vi "XY_plot_gnuplot.vi"(0 "Plot Array":cluster{dbl[], dbl[]}[](array[cluster])=[{[500.0, 500.0, 953.54, 215.0, 270.0, 320.0, 445.0, 525.0, 600.0, 675.0, 750.0, 825.0, 900.0, 960.0, 1010.0, 1060.0], [4.614524, 4.54365, 5.818368, 0.1374656, 0.6662545, 1.465458, 3.619824, 4.848976, 5.887329, 5.940571, 6.152151, 5.717487, 5.600293, 5.40069, 5.154843, 5.121789]}, {[100.0, 150.0, 215.0, 270.0, 320.0, 445.0, 525.0, 600.0, 675.0, 750.0, 825.0, 900.0, 960.0, 1010.0, 1060.0], [0.002314715, -0.00693192, 0.120417, 0.6880509, 1.519176, 3.513709, 5.065183, 6.116033, 6.096773, 5.938465, 5.593788, 5.5597, 5.387002, 5.304077, 4.887903]}] {"?" format="%.2f"; "?" format="%.2f"}, 1 "Job Directory":path=path "/G4_2_HD/Users/paulhayden/Documents/Projects/Westlakes_resolution") -> (2 "Saved Automatically?":bool, 3 "Tex Info String":string="set term epslatex\nset output \"Plot.eps\"\nset xlabel '$Distance~(m)$'\nset ylabel '$DF~(s/m^3)\\times10^6$'\nset samples 1000\nset pointsize 1.00\nset title '$B38~Centreline~Glc$' 0, 0\nset size 0.75,0.9\n\n#set key 450, -2.5833\n unset key\nset label 1 '~~~~~~~~~~~Angle~(deg)~=~0' at -100, -2.58\nset label 2 '~~~~~~~~~~~Height~(m)~=~5' at -100, -3.27\n set xrange [0 : 500] \n# set autoscale x \n set yrange [0.10000 : 7]\n# set autoscale y \n\nplot \"B38_Centreline_Glc.dat\" index 0 using 1:2 axes x1y1 title '$File=B38R~DDD.xls$' with points 1 1, \\\n\"B38_Centreline_Glc.dat\" index 1 using 1:2 axes x1y1 title '$File=B38R~DDD~1.xls$' with points 1 3", 4 "Plot data file":path)   [LabVIEW 2012]
uses:
  Gnuplot_Label.ctl
  gnuplotScriptComponents/gridlines.ctl
  gnuplotScriptComponents/legendProperties.ctl
  gnuplotScriptComponents/legendAppearance.ctl
  gnuplotScriptComponents/alignment.ctl
  gnuplotScriptComponents/at.ctl
  Results_plotter_Global.vi
  <vilib>/Analysis/baseanly.llb/Mean (DBL).vi
  <vilib>/Analysis/NI_AALBase.lvlib
  <vilib>/Analysis/NI_AALPro.lvlib
panel:
  in  "Call GNUPLOT":bool
  in  "Show Re-Run Gnuplot?":bool
  in  "Tab Control":T1(tab)
  in  "Plot Title":u16(ring) items=["Title String Only", "Number of Measurements", "WD::", "Pt::", "U0:W:", "U1:W:", "U2:W:l", "U2:W:u", "U3:W:", "U4:W:", "U0:E:", "U1:E:", "U2:E:l", "U2:E:u", "U3:E:", "U4:E:", "U2_{tower}::", "U3_{tower}::", "U4_{tower}::", "U3W/U3_{tower}::", "U3E/U3_{tower}::", "U4W/U4_{tower}::", "U4E/U4_{tower}::", "U0W/U4W::", "U0E/U4E::", "$U0W/U4_{tower}$::", "$U0E/U4_{tower}$::", "U2Wl/U2_{tower}::", "U2Wu/U2_{tower}::", "U2El/U2_{tower}::", "U2Eu/U2_{tower}::"]
  in  "Plot Title":string
  in  "Added labels":i32[](listbox)
  in  "Show Labels?":bool
  in  "Summarise":u16(ring) items=["All Series", "U2Wl/U2_{tower}__Pt=1__", "U2Wl/U2_{tower}__Pt=2__", "U2Wl/U2_{tower}__Pt=3__", "U2Wl/U2_{tower}__Pt=4__", "U2Wu/U2_{tower}__Pt=1__", "U2Wu/U2_{tower}__Pt=2__", "U2Wu/U2_{tower}__Pt=3__", "U2Wu/U2_{tower}__Pt=4__"]
  in  "X Log?":bool
  in  "Y Log?":bool
  in  "Ymin Val":dbl
  in  "Ymin":bool=TRUE
  in  "Xmin Val":dbl
  in  "Xmin":bool=TRUE
  in  "Xmax Val":dbl
  in  "Xmax":bool=TRUE
  in  "Ymax Val":dbl
  in  "Ymax":bool=TRUE
  in  "Major Gridlines":T2
  in  "Minor Gridlines":T2
  out "Time format?":bool
  in  "precision":string
  out "Profile offset":dbl
  in  "Offset?":bool
  in  "Mode":T3
  in  "Separation":dbl=1.2
  in  "Fit type":T4(ring)
  in  "Put Coeff\nin Results file":bool
  in  "Analysis":T5(ring)
  in  "Wavelength?":bool
  in  "Auto Zp":bool=TRUE
  in  "Fixed Zp":dbl format="%.2f"
  in  "Something about fit..!":bool
  in  "Black and white?":bool
  in  "plot error bars?":bool
  in  "Plot style":u16[](array[ring])=[0, 0, 0, 0, 0, 0, 0, 0, 0, 0, 0] items=["points", "lines", "linespoints"]
  in  "Point Size":dbl=1.2 format="%.2f"
  in  "Graph Height":string="0.9"
  in  "Graph width":string="0.75"
  in  "Show legend?":bool
  in  "Legend Position":u16(ring) items=["LabVIEW calculated", "top left", "top right", "bottom left", "bottom right", "below"]
  in  "Reverse order":bool
  in  "Save data analysis file":bool
  out "Path":path
  in  "Filename Max length":i32=28
  out "With legend":i32=580
  out "No Legend":i32=397
  out "No of Series":i32=2
  out "X location":dbl=-100.0
  out "Y location":dbl=-2.583333333333333
  out "Delta y":dbl=0.6900000000000001
  out "Extra range":dbl
  out "Final Title":string="B38 Centreline Glc"
  out "XY Graph":cluster{dbl[], dbl[]}[](graph)=[{[215.0, 270.0, 320.0, 445.0, 500.0, 500.0, 525.0, 600.0, 675.0, 750.0, 825.0, 900.0, 953.54, 960.0, 1010.0, 1060.0], [0.1374656, 0.6662545, 1.465458, 3.619824, 4.614524, 4.54365, 4.848976, 5.887329, 5.940571, 6.152151, 5.717487, 5.600293, 5.818368, 5.40069, 5.154843, 5.121789]}, {[100.0, 150.0, 215.0, 270.0, 320.0, 445.0, 525.0, 600.0, 675.0, 750.0, 825.0, 900.0, 960.0, 1010.0, 1060.0], [0.002314715, -0.00693192, 0.120417, 0.6880509, 1.519176, 3.513709, 5.065183, 6.116033, 6.096773, 5.938465, 5.593788, 5.5597, 5.387002, 5.304077, 4.887903]}]
  # "Scales"
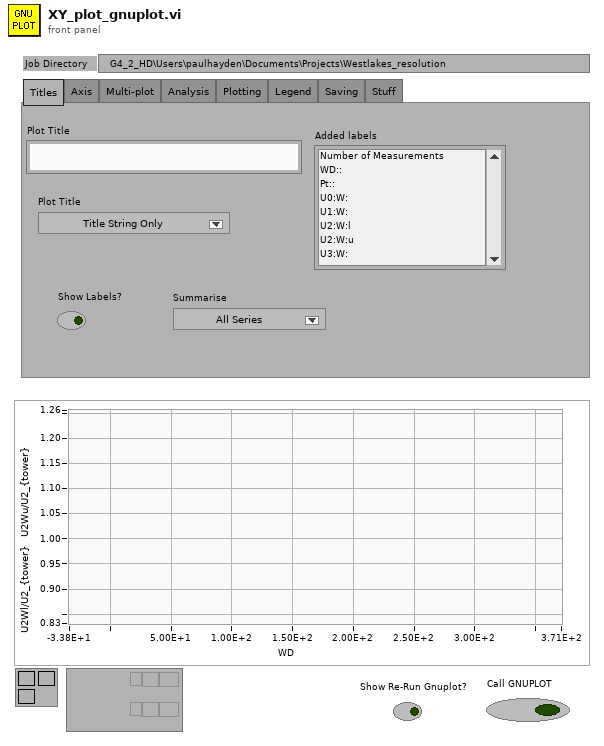
[diagram p1: front panel]
types:
  T1 = enum32{"Titles", "Axis", "Multi-plot", "Analysis", "Plotting", "Legend", "Saving", "Stuff"}
  T2 = typedef "gridlines.ctl" = enum16{"None", "X only", "Y only", "Both X and Y"}
  T3 = typedef "Gnuplot_Label.ctl" = enum16{"3 Labels per plot", "Only Center label", "Only Bottom Label"}
  T4 = enum16{"None", "Spline", "Linear", "2nd Poly", "3rd Poly", "4th Poly", "Gauss Lat", "Gauss vert", "Gauss Vert with 2 sig", "Guass glc"}
  T5 = enum16{"None", "% change", "Spectrum", "Norm Spec"}
  T6 = enum16{"None", "Lines", "Linespoints", "Spline", "Linear", "2nd Ploy", "3rd Poly", "4th Poly", "Gauss Lat", "Gauss vert", "Guass glc"}
  T7 = cluster{"Output":dbl[], "PercentageDifferenceArray":dbl[]}[]
  T8 = cluster{"Output":dbl[], "PercentageDifferenceArray":dbl[]}
  T9 = typedef "legendProperties.ctl" = cluster{"Appearance":T10, "Alignment":T11, "Location":string, "\"At\" location":T12}
  T10 = typedef "legendAppearance.ctl" = cluster{"layout":string, "text-sample order":string, "key order":string, "surroundingBox":string}
  T11 = typedef "alignment.ctl" = cluster{"Horizontal":string, "Vertical":string}
  T12 = typedef "at.ctl" = cluster{"XcoordSys":string, "YcoordSys":string, "Xvalue":dbl, "Yvalue":dbl}
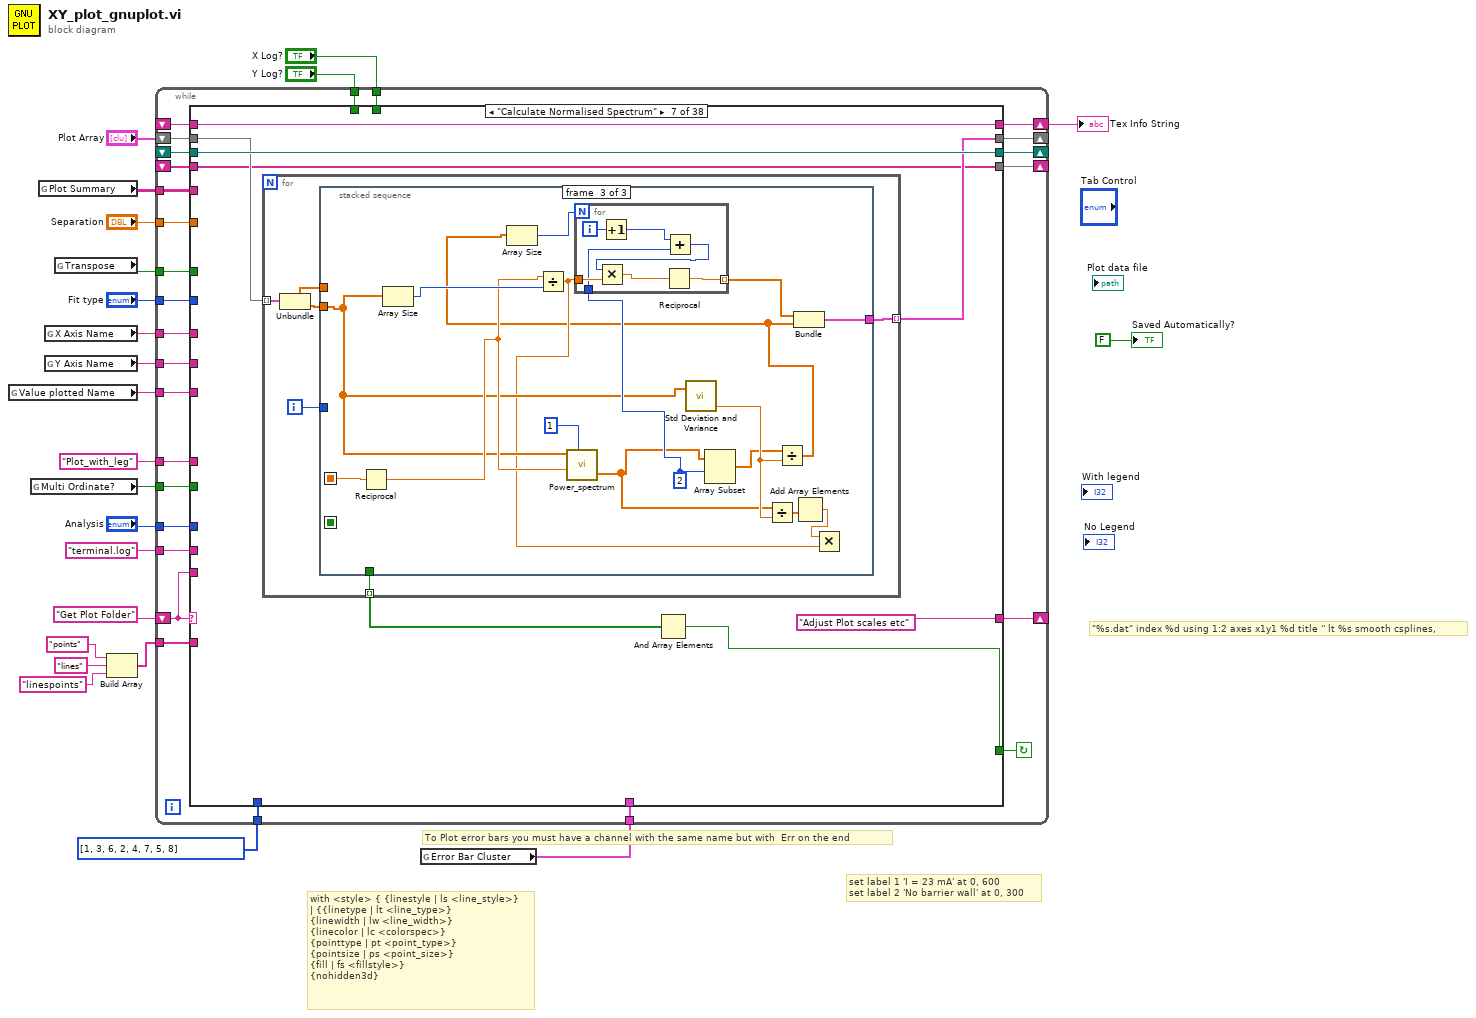
[diagram p0: block diagram]
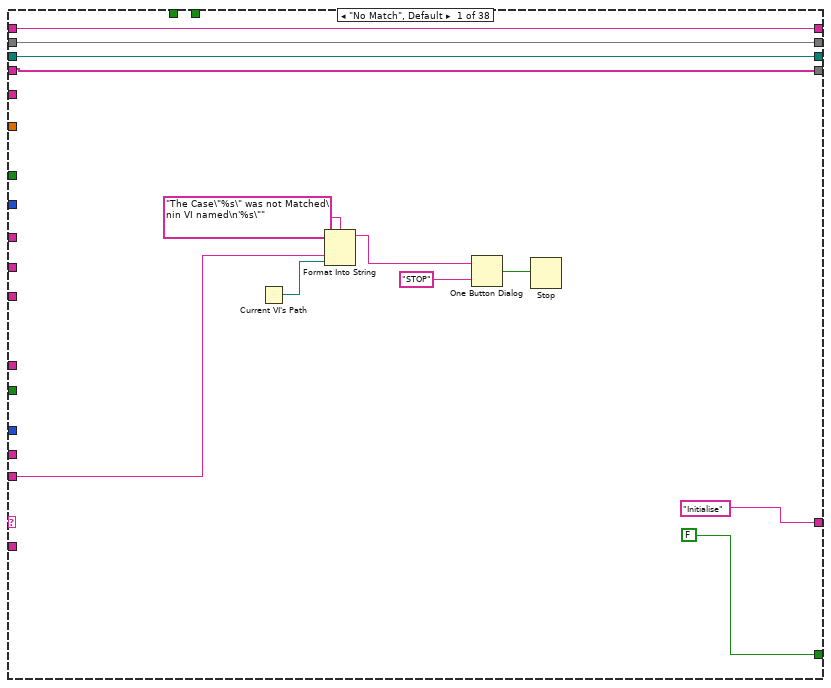
[diagram p2: hidden frame]
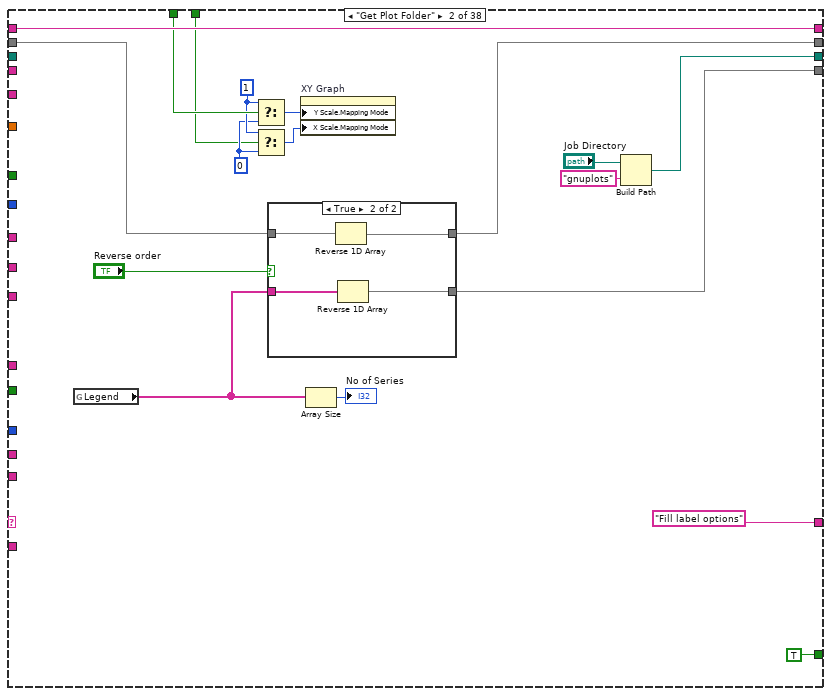
[diagram p3: hidden frame]
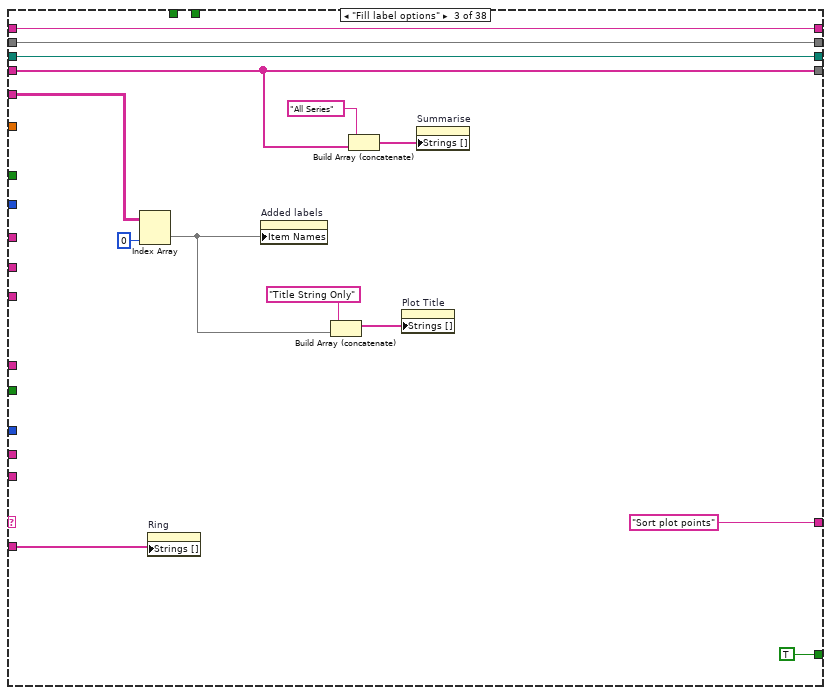
[diagram p5: hidden frame]
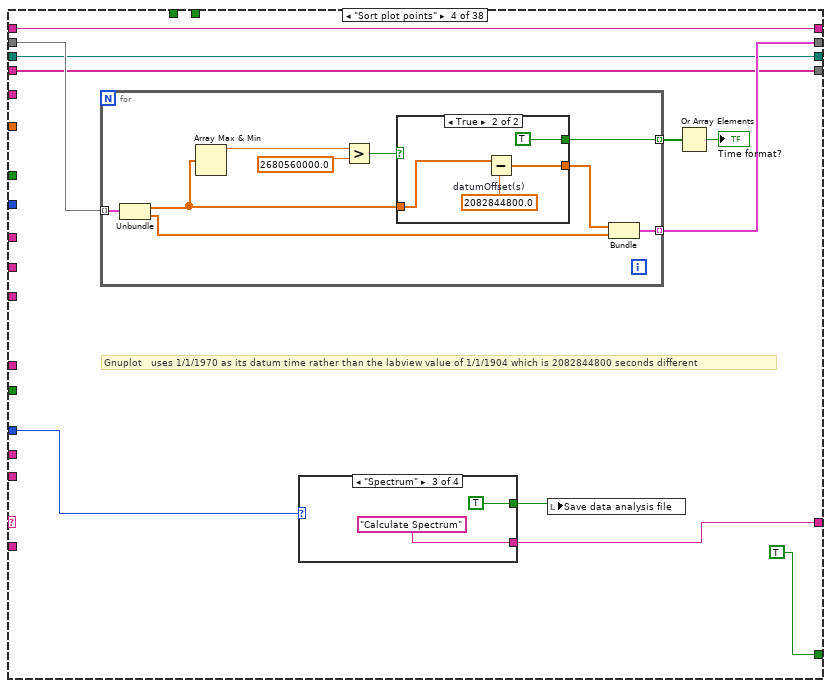
[diagram p6: hidden frame]
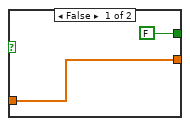
[diagram p7: hidden frame]
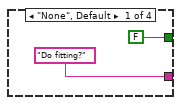
[diagram p8: hidden frame]
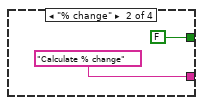
[diagram p9: hidden frame]
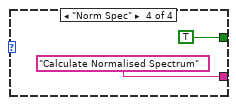
[diagram p10: hidden frame]
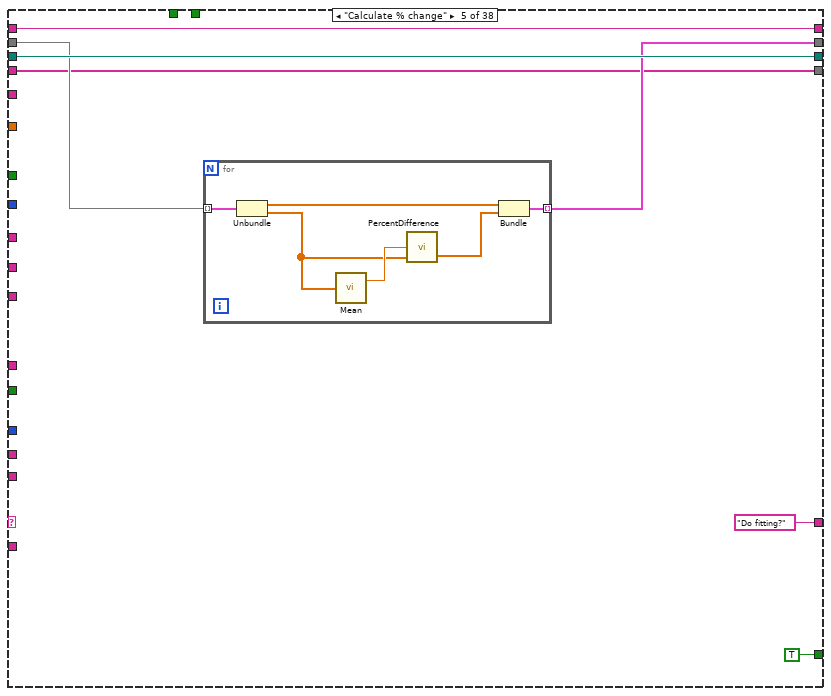
[diagram p11: hidden frame]
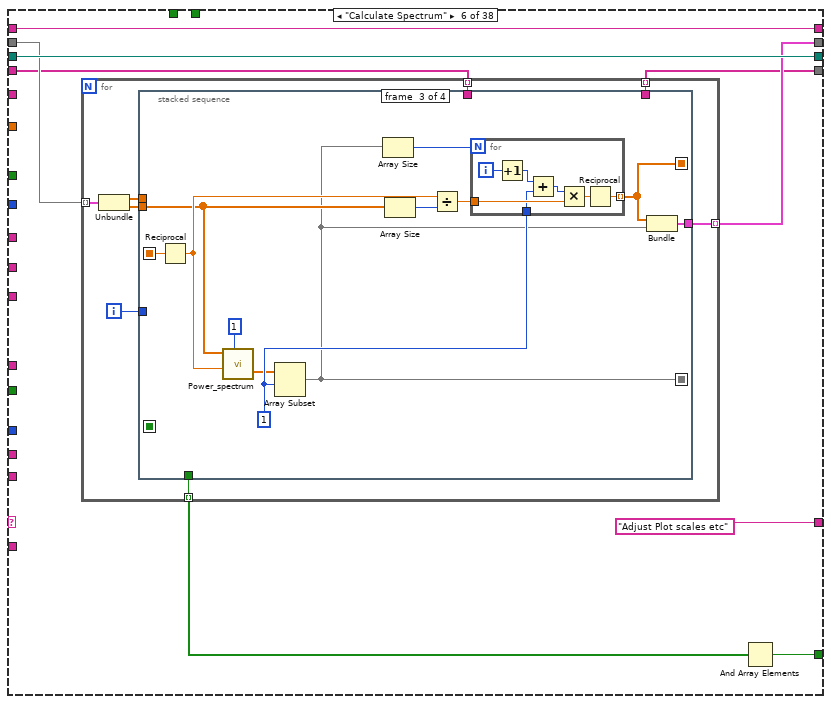
[diagram p12: hidden frame]
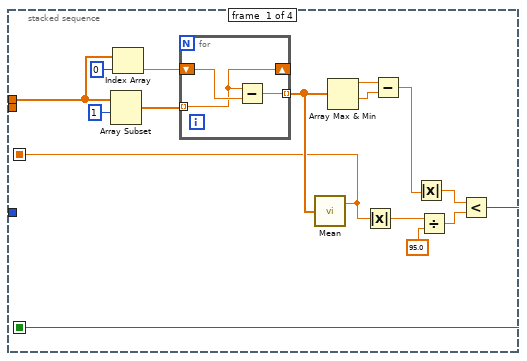
[diagram p13: hidden frame]
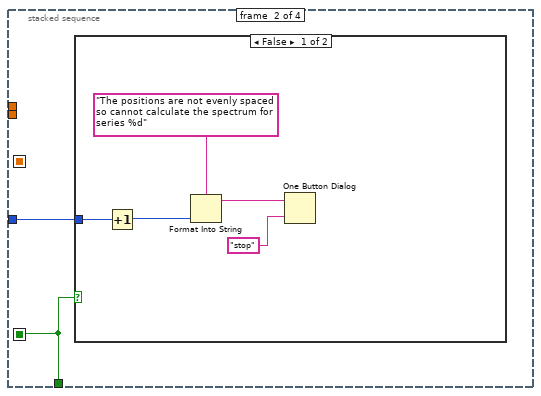
[diagram p14: hidden frame]
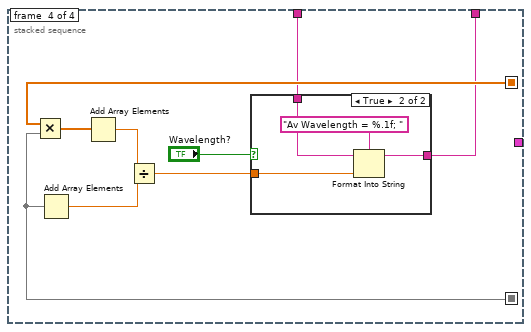
[diagram p16: hidden frame]
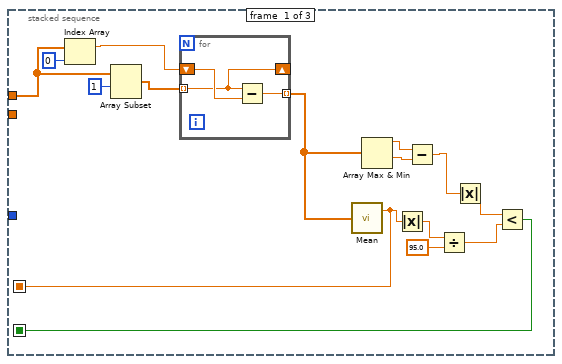
[diagram p18: hidden frame]
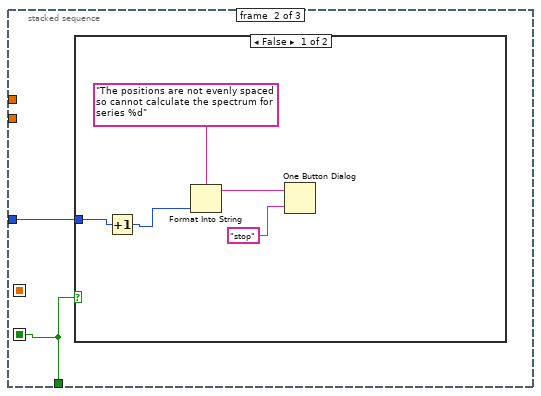
[diagram p19: hidden frame]
diagram:
  # "\"%s.dat\" index %d using 1:2 axes x1y1 %d title '' lt %s smooth csplines,"
  # "with <style> { {linestyle | ls <line_style>} \n| {{linetype | lt <line_type>} \n{linewidth | lw <line_width>} \n{linecolor | lc <colorspec>} \n{pointtype | pt <point_type>} \n{pointsize | ps <point_size>} \n{fill | fs <fillstyle>} \n{nohidden3d}"
  # "To Plot error bars you must have a channel with the same name but with  Err on the end"
  # "set label 1 'I = 23 mA' at 0, 600\nset label 2 'No barrier wall' at 0, 300"
  n1 = global read "Results_plotter_Global.vi" "Value plotted Name"() -> (w19:string)
  n2 = global read "Results_plotter_Global.vi" "Multi Ordinate?"() -> (w1:bool)
  n3 = global read "Results_plotter_Global.vi" "Plot Summary"() -> (w22:string[][])
  n4 = global read "Results_plotter_Global.vi" "X Axis Name"() -> (w21:string)
  n5 = global read "Results_plotter_Global.vi" "Y Axis Name"() -> (w20:string)
  n6 = global read "Results_plotter_Global.vi" "Transpose"() -> (w2:bool)
  n7 = Build Array("points", "lines", "linespoints") -> (w9:string[])
  n8 = global read "Results_plotter_Global.vi" "Error Bar Cluster"() -> (w4:cluster{string[]}[])
  n9 = while {
    shift-left: "Get Plot Folder" -> [w48]
    shift-right: [w49] -> _
    tunnel: w22 -> [w47]
    shift-right: [w46] -> _
    shift-left: _ -> [w45]
    tunnel: "Analysis" -> [w44]
    tunnel: w21 -> [w43]
    tunnel: w20 -> [w42]
    tunnel: w19 -> [w41]
    shift-right: [w39] -> _
    shift-left: "Plot Array" -> [w40]
    shift-right: [w37] -> w17
    shift-left: _ -> [w38]
    tunnel: "Plot_with_leg" ("name or relative path") -> [w36]
    tunnel: "Fit type" -> [w35]
    shift-right: [w34] -> _
    shift-left: _ -> [w33]
    tunnel: "terminal.log" -> [w32]
    tunnel: w9 -> [w31]
    tunnel: i32[] [1, 3, 6, 2, 4, 7, 5, 8] ("Plot style") -> [w30]
    tunnel: "Separation" -> [w29]
    tunnel: "Y Log?" -> [w28]
    tunnel: w4 -> [w27]
    tunnel: "X Log?" -> [w26]
    tunnel: w2 -> [w25]
    tunnel: w1 -> [w24]
    stop <- w50 continue-if-true
    n10 = case shown="\"Calculate Normalised Spectrum\"" w48 {
      tunnel: [FALSE TRUE TRUE ("Top Level") TRUE TRUE w150 w223 TRUE TRUE TRUE ("Top Level") TRUE ("Top Level") TRUE ("Top Level") TRUE ("Top Level") TRUE ("Top Level") TRUE ("Top Level") TRUE ("Top Level") TRUE ("Top Level") TRUE ("Top Level") TRUE ("Top Level") "Call GNUPLOT" w676 w749 TRUE ("Top Level") TRUE ("Top Level") TRUE ("Top Level") TRUE ("Top Level") TRUE ("Top Level") TRUE ("Top Level") TRUE ("Top Level") TRUE ("Top Level") TRUE ("Top Level") TRUE ("Top Level") TRUE ("Top Level") TRUE ("Top Level") TRUE ("Top Level") w1575 FALSE ("Top Level") FALSE ("Top Level")] -> w50
      tunnel: ["Initialise" "Fill label options" "Sort plot points" w104 "Do fitting?" "Adjust Plot scales etc" "Adjust Plot scales etc" "Adjust Plot scales etc" "Add fitted line styles" "Adjust Plot scales etc" w381 "Fill Second legend" "Fill Second legend" "Fill Second legend" "Calculate plot max and min values" "Sort out plot title" w566 w635 "Create plot directory" w659 w675 w748 w892 "Edit Legend names" w1076 "Labels?" ("t") "Labels?" ("t") w1237 w1248 "Plot Command" "Write gnuplot file" ("t") "Execute shell script" ("t") "Has pdf been generated?" ("t") w1552 "Input Fit Coefficients into results file?" "Read Fit Coefficients" ("t") "End" ("t") "End" ("t")] -> w49
      tunnel: w48 -> [w57 _ _ _ _ _ _ _ _ _ _ _ _ _ _ _ _ _ _ _ _ _ _ _ _ _ _ _ _ _ _ _ _ _ _ _ _ _]
      tunnel: w47 -> [_ _ w100 _ _ _ _ _ _ _ _ _ _ _ _ _ w575 _ _ _ w674 w747 _ _ _ _ _ _ w1247 _ _ _ _ _ _ _ _ _]
      tunnel: [w54 w77 w94 w108 w139 w155 w229 w290 w305 w366 w391 w417 w426 w438 w465 w499 w568 w636 w647 w661 w677 w750 w904 w944 w1091 w1158 w1214 w1244 w1254 w1378 w1409 w1537 w1545 w1558 w1569 w1580 w1598 w1673] -> w46
      tunnel: w45 -> [w54 _ w94 w108 w139 w155 w229 w290 w305 w366 w391 w417 w426 w438 w461 w499 w567 w632 w648 w656 w677 w750 w904 w944 w1091 w1158 w1214 w1244 w1254 w1378 w1409 w1537 w1545 w1558 w1569 w1580 w1598 w1673]
      tunnel: w44 -> [_ _ _ w105 _ _ _ _ _ _ w382 _ _ w432 _ _ _ w623 _ _ w670 w742 w901 _ _ _ _ _ _ _ _ _ _ _ _ _ _ _]
      tunnel: w43 -> [_ _ _ _ _ _ _ _ w296 _ _ w413 w425 _ _ _ _ _ _ _ w673 w746 w899 _ _ _ _ _ _ _ _ _ _ _ _ _ _ _]
      tunnel: w42 -> [_ _ _ _ _ _ _ _ w295 _ _ w412 w424 w437 _ _ _ _ _ _ w672 w745 w900 _ _ _ _ _ _ _ _ _ _ _ _ _ _ _]
      tunnel: w41 -> [_ _ _ _ _ _ _ _ _ _ _ _ _ _ _ _ _ _ _ _ w669 _ _ _ _ _ _ _ _ _ _ _ _ _ _ _ w1592 _]
      tunnel: w40 -> [w53 w72 w95 w110 w138 w154 w228 w286 w301 w365 w380 w416 w423 w436 w464 w496 w581 w634 w651 w664 w668 w744 w905 w931 w1086 w1153 w1210 w1241 w1249 w1379 w1410 w1543 w1550 w1565 w1574 w1584 w1587 w1678]
      tunnel: [w53 w71 w95 w109 w137 w153 w227 w286 w294 w365 w380 w416 w423 w436 w464 w496 w581 w634 w651 w664 w668 w741 w905 w931 w1086 w1153 w1210 w1241 w1249 w1379 w1410 w1543 w1550 w1565 w1574 w1584 w1587 w1678] -> w39
      tunnel: w38 -> [w52 w76 w96 w107 w136 w152 w226 w289 w304 w363 w383 w415 w422 w435 w463 w500 w576 w633 w650 w663 w678 w751 _ w942 w1090 w1124 w1190 w1232 w1251 w1375 w1407 w1532 w1548 w1563 w1572 w1582 w1601 w1676]
      tunnel: [w52 w76 w96 w107 w136 w152 w226 w289 w304 w363 w383 w415 w422 w435 w463 w500 w576 w633 w650 w663 w678 w751 w895 w940 w1090 w1121 w1189 w1231 w1252 w1371 w1406 w1532 w1548 w1563 w1572 w1582 w1601 w1676] -> w37
      tunnel: w36 -> [_ _ _ _ _ _ _ _ _ _ _ _ _ _ _ _ _ _ _ _ _ _ _ _ _ _ _ _ _ _ _ _ _ _ _ _ _ _]
      tunnel: w35 -> [_ _ _ _ _ _ _ w287 w303 _ w385 _ _ _ _ _ _ _ _ _ _ _ w893 w946 _ _ _ _ _ w1344 w1403 _ _ _ _ w1579 w1594 _]
      tunnel: [w51 w70 w92 w106 w135 w148 w225 w288 w298 w362 w387 w414 w421 w434 w462 w498 w580 w631 w649 w662 w671 w743 w903 w947 w1092 w1157 w1213 w1243 w1253 w1365 w1408 w1538 w1549 w1564 w1573 w1583 w1602 w1677] -> w34
      tunnel: w33 -> [w51 _ w92 w106 w135 w149 w225 w288 w299 w362 w387 w414 w421 w434 w462 w498 w580 w631 w649 w662 w671 w743 w903 w947 w1093 w1157 w1213 w1243 w1253 w1365 w1408 w1538 w1549 w1564 w1573 w1583 w1602 w1677]
      tunnel: w32 -> [_ _ _ _ _ _ _ _ _ _ _ _ _ _ _ _ _ _ _ _ _ _ _ _ _ _ _ _ _ _ _ _ w1544 _ _ _ _ w1671]
      tunnel: w31 -> [_ _ w90 _ _ _ _ _ _ _ _ _ _ _ _ _ _ _ _ _ _ _ _ _ _ _ _ _ _ _ _ _ _ _ _ _ _ _]
      tunnel: w30 -> [_ _ _ _ _ _ _ _ _ _ _ _ _ _ _ _ _ _ _ _ _ _ _ _ _ _ _ _ _ _ w1401 w1534 _ _ _ _ _ _]
      tunnel: w29 -> [_ _ _ _ _ _ _ _ _ _ _ _ _ _ _ _ _ _ _ _ _ w740 _ _ w1085 _ _ _ _ w1362 _ _ _ _ _ _ _ _]
      tunnel: w28 -> [_ w69 _ _ _ _ _ _ _ _ _ _ _ _ _ _ _ _ _ _ _ _ _ _ _ w1137 w1201 _ w1246 w1359 _ _ _ _ _ _ _ _]
      tunnel: w27 -> [_ _ _ _ _ _ _ _ _ _ _ _ _ _ _ w469 _ _ _ _ _ w739 _ _ _ _ _ _ _ _ w1400 _ _ _ _ _ _ _]
      tunnel: w26 -> [_ w64 _ _ _ _ _ _ _ _ _ _ _ _ _ _ _ _ _ _ _ _ _ _ _ w1134 _ _ w1245 w1354 _ _ _ _ _ _ _ _]
      tunnel: w25 -> [_ _ _ _ _ _ _ _ _ _ _ _ _ _ _ w467 _ _ _ _ _ w738 _ w932 _ _ _ _ _ w1349 w1397 _ _ _ _ _ _ _]
      tunnel: w24 -> [_ _ _ _ _ _ _ _ _ _ _ _ _ _ _ _ _ _ _ _ _ _ _ _ _ _ _ _ _ _ _ _ _ _ _ _ _ _]
      frame "No Match", Default {
        n11 = Current VI's Path() -> (path=w56:path)
        n12 = Format Into String(format string="The Case\"%s\" was not Matched\nin VI named\n'%s\"" ("Format String"), w57, w56) -> (resulting string=w60:string)  [unwired: 2 in, 1 out]
        n13 = One Button Dialog(message=w60, button name ("OK")="STOP") -> (true=w58:bool)
        n14 = Stop(stop? (T)=w58) -> ()
      }
      frame "Get Plot Folder" {
        w65 = u8 0 ("f")
        w66 = u8 1 ("Y Scale.Mapping Mode")
        n15 = global read "Results_plotter_Global.vi" "Legend"() -> (w63:string[])
        n16 = Select(t=w66, s=w69, f=w65) -> (s? t:f=w68:u8)
        n17 = Select(t=w66, s=w64, f=w65) -> (s? t:f=w67:u8)
        n18 = case shown="True" "Reverse order" {
          tunnel: w72 -> [w82 w86]
          tunnel: [w82 w85] -> w71
          tunnel: w63 -> [w81 w84]
          tunnel: [w81 w83] -> w70
          frame False {
          }
          frame True {
            n19 = Reverse 1D Array(array=w86) -> (reversed array=w85:T7)
            n20 = Reverse 1D Array(array=w84) -> (reversed array=w83:string[])
          }
        }
        n21 = property on="XY Graph" class="XYGraph (strict)"("Y Scale.Mapping Mode"=w68, "X Scale.Mapping Mode"=w67) -> ()  [unwired: 2 in, 2 out]
        n22 = Array Size(array=w63) -> (size(s)=→"No of Series":i32)
        n23 = Build Path(base path="Job Directory", name or relative path="gnuplots") -> (appended path=w77:path)
      }
      frame "Fill label options" {
        n24 = Index Array(array=w100, index (col)=0 ("disabled index (col)")) -> (element=w88:string[])  [unwired: 1 in]
        n25 = property on="Ring" class="Ring (strict)"("Strings []"=w90) -> ()  [unwired: 2 in, 2 out]
        n26 = property on="Added labels" class="LstBox (strict)"("Item Names"=w88) -> ()  [unwired: 2 in, 2 out]
        n27 = Build Array (concatenate)("Title String Only", w88) -> (w87:string[])
        n28 = Build Array (concatenate)("All Series", w92) -> (w93:string[])
        n29 = property on="Plot Title" class="Ring (strict)"("Strings []"=w87) -> ()  [unwired: 2 in, 2 out]
        n30 = property on="Summarise" class="Ring (strict)"("Strings []"=w93) -> ()  [unwired: 2 in, 2 out]
      }
      frame "Sort plot points" {
        # "Gnuplot   uses 1/1/1970 as its datum time rather than the labview value of 1/1/1904 which is 2082844800 seconds different"
        n31 = for {
          tunnel: w110 -> [w119] mode=indexing
          tunnel: [w120] -> w109 mode=indexing
          tunnel: [w112] -> w102 mode=indexing
          n32 = Unbundle(w119) -> ("Output"=w115:dbl[], "PercentageDifferenceArray"=w116:dbl[])
          n33 = Array Max & Min(array=w115) -> (max value=w118:dbl)  [unwired: 3 out]
          n34 = Greater?(x=w118, y=2680560000.0) -> (0:w113:bool)
          n35 = case shown="True" w113 {
            tunnel: w115 -> [w122 w126]
            tunnel: [w122 w124] -> w114
            tunnel: [FALSE TRUE] -> w112
            frame False {
            }
            frame True {
              w125 = 2082844800.0  # datumOffset(s)
              n36 = Subtract(x=w126, y=w125) -> (x-y=w124:dbl[])
            }
          }
          n37 = Bundle("Output"=w114, "PercentageDifferenceArray"=w116) -> (w120:T8)  [unwired: 1 out]
        }
        n38 = case shown="\"Spectrum\"" w105 {
          tunnel: ["Do fitting?" "Calculate % change" "Calculate Spectrum" "Calculate Normalised Spectrum"] -> w104
          tunnel: [FALSE ("Save data analysis file") FALSE ("Save data analysis file") TRUE ("Save data analysis file") TRUE ("Save data analysis file")] -> w103
          frame "None", Default {
          }
          frame "% change" {
          }
          frame "Spectrum" {
          }
          frame "Norm Spec" {
          }
        }
        n39 = local write "Save data analysis file"(w103) -> ()
        n40 = Or Array Elements(Boolean array=w102) -> (logical OR=→"Time format?":bool)
      }
      frame "Calculate % change" {
        n41 = for {
          tunnel: w138 -> [w147] mode=indexing
          tunnel: [w145] -> w137 mode=indexing
          n42 = Unbundle(w147) -> ("Output"=w146:dbl[], "PercentageDifferenceArray"=w143:dbl[])
          n43 = call-poly <vilib>:"Mean.vi"("X"=w143) -> ("mean"=w144:dbl)  [unwired: 1 out]
          n44 = call "PercentDifference.vi"("CompareeArray"=w143, "Basis"=w144) -> ("PercentageDifferenceArray"=w142:dbl[])  [unwired: 1 in, 1 out]
          n45 = Bundle("Output"=w146, "PercentageDifferenceArray"=w142) -> (w145:T8)  [unwired: 1 out]
        }
      }
      frame "Calculate Spectrum" {
        n46 = for {
          tunnel: w154 -> [w163] mode=indexing
          tunnel: [w164] -> w153 mode=indexing
          tunnel: [w159] -> w151 mode=indexing
          tunnel: w149 -> [w158] mode=indexing
          tunnel: [w157] -> w148 mode=indexing
          i -> [w160]
          n47 = Unbundle(w163) -> ("Output"=w161:dbl[], "PercentageDifferenceArray"=w162:dbl[])
          n48 = stacked-sequence {
            seq-local: [w166 _ _ _] -> [_ _ w196 _]
            seq-local: [w165 _ _ _] -> [_ w183 _ _]
            seq-local: [_ _ w191 _] -> [_ _ _ w216]
            seq-local: [_ _ w190 _] -> [_ _ _ w217]
            tunnel: [_ _ w201 _] -> w164
            tunnel: w162 -> [_ _ w194 _]
            tunnel: w161 -> [w177 _ _ _]
            tunnel: w160 -> [_ w184 _ _]
            tunnel: [_ w183 _ _] -> w159
            tunnel: w158 -> [_ _ _ w212]
            tunnel: [_ _ _ w210] -> w157
            frame #0 {
              n49 = Array Subset(array=w177, index=1) -> (w175:dbl[])  [unwired: 1 in]
              n50 = Index Array(array=w177, index=0) -> (element=w176:dbl)
              n51 = for {
                shift-right: [w181] -> _
                shift-left: w176 -> [w182]
                tunnel: w175 -> [w181] mode=indexing
                tunnel: [w180] -> w172 mode=indexing
                n52 = Subtract(x=w181, y=w182) -> (x-y=w180:dbl)
              }
              n53 = call-poly <vilib>:"Mean.vi"("X"=w172) -> ("mean"=w166:dbl)  [unwired: 1 out]
              n54 = Array Max & Min(array=w172) -> (max value=w174:dbl, min value=w173:dbl)  [unwired: 2 out]
              n55 = Absolute Value(x=w166) -> (abs(x)=w169:dbl)
              n56 = Subtract(x=w174, y=w173) -> (x-y=w171:dbl)
              n57 = Absolute Value(x=w171) -> (abs(x)=w170:dbl)
              n58 = Divide(x=w169, y=95.0) -> (x/y=w167:dbl)
              n59 = Less?(x=w170, y=w167) -> (x < y?=w165:bool)
            }
            frame #1 {
              n60 = case shown="False" w183 {
                tunnel: w184 -> [w189 _]
                frame False {
                  n61 = Increment(x=w189) -> (x+1=w188:i32)
                  n62 = Format Into String(format string="The positions are not evenly spaced so cannot calculate the spectrum for series %d", w188) -> (resulting string=w186:string)  [unwired: 2 in, 1 out]
                  n63 = One Button Dialog(message=w186, button name ("OK")="stop") -> ()  [unwired: 1 out]
                }
                frame True {
                }
              }
            }
            frame #2 {
              w197 = 1 ("index")
              n64 = Reciprocal(x=w196) -> (1/x=w195:dbl)
              n65 = call "Power_spectrum.vi"("U"=w194, "Sampling frequency"=w195, "Block No"=1) -> ("Spectrum output array"=w193:dbl[])  [unwired: 1 in, 2 out]
              n66 = Array Subset(array=w193, index=w197) -> (w190:dbl[])  [unwired: 1 in]
              n67 = Array Size(array=w190) -> (size(s)=w200:i32)
              n68 = Array Size(array=w194) -> (size(s)=w198:i32)
              n69 = Divide(x=w195, y=w198) -> (x/y=w192:dbl)
              n70 = for {
                N: w200 -> [_]
                tunnel: [w205] -> w191 mode=indexing
                tunnel: w192 -> [w207]
                tunnel: w197 -> [w203]
                i -> [w208]
                n71 = Increment(x=w208) -> (x+1=w204:i32)
                n72 = Add(x=w204, y=w203) -> (x+y=w202:i32)
                n73 = Multiply(x=w202, y=w207) -> (x*y=w206:dbl)
                n74 = Reciprocal(x=w206) -> (1/x=w205:dbl)
              }
              n75 = Bundle(w191, w190) -> (w201:cluster{dbl[], dbl[]})  [unwired: 1 out]
            }
            frame #3 {
              n76 = Multiply(x=w216, y=w217) -> (x*y=w215:dbl[])
              n77 = Add Array Elements(numeric array=w217) -> (sum=w213:dbl)
              n78 = Add Array Elements(numeric array=w215) -> (sum=w214:dbl)
              n79 = Divide(x=w214, y=w213) -> (x/y=w211:dbl)
              n80 = case shown="True" "Wavelength?" {
                tunnel: w212 -> [w218 w222]
                tunnel: w211 -> [_ w221]
                tunnel: [w218 w219] -> w210
                frame False {
                }
                frame True {
                  n81 = Format Into String(format string="Av Wavelength = %.1f; ", initial string=w222, w221) -> (resulting string=w219:string)  [unwired: 1 in, 1 out]
                }
              }
            }
          }
        }
        n82 = And Array Elements(Boolean array=w151) -> (logical AND=w150:bool)
      }
      frame "Calculate Normalised Spectrum" {
        n83 = for {
          tunnel: w228 -> [w235] mode=indexing
          tunnel: [w236] -> w227 mode=indexing
          tunnel: [w231] -> w224 mode=indexing
          i -> [w232]
          n84 = Unbundle(w235) -> ("Output"=w233:dbl[], "PercentageDifferenceArray"=w234:dbl[])
          n85 = stacked-sequence {
            seq-local: [w238 _ _] -> [_ _ w271]
            seq-local: [w237 _ _] -> [_ w255 _]
            tunnel: [_ _ w277] -> w236
            tunnel: w234 -> [_ _ w269]
            tunnel: w233 -> [w249 _ _]
            tunnel: w232 -> [_ w256 _]
            tunnel: [_ w255 _] -> w231
            frame #0 {
              n86 = Index Array(array=w249, index=0) -> (element=w248:dbl)
              n87 = Array Subset(array=w249, index=1) -> (w247:dbl[])  [unwired: 1 in]
              n88 = for {
                shift-right: [w253] -> _
                shift-left: w248 -> [w254]
                tunnel: w247 -> [w253] mode=indexing
                tunnel: [w252] -> w244 mode=indexing
                n89 = Subtract(x=w253, y=w254) -> (x-y=w252:dbl)
              }
              n90 = call-poly <vilib>:"Mean.vi"("X"=w244) -> ("mean"=w238:dbl)  [unwired: 1 out]
              n91 = Array Max & Min(array=w244) -> (max value=w246:dbl, min value=w245:dbl)  [unwired: 2 out]
              n92 = Absolute Value(x=w238) -> (abs(x)=w241:dbl)
              n93 = Subtract(x=w246, y=w245) -> (x-y=w243:dbl)
              n94 = Divide(x=w241, y=95.0) -> (x/y=w239:dbl)
              n95 = Absolute Value(x=w243) -> (abs(x)=w242:dbl)
              n96 = Less?(x=w242, y=w239) -> (x < y?=w237:bool)
            }
            frame #1 {
              n97 = case shown="False" w255 {
                tunnel: w256 -> [w261 _]
                frame False {
                  n98 = Increment(x=w261) -> (x+1=w260:i32)
                  n99 = Format Into String(format string="The positions are not evenly spaced so cannot calculate the spectrum for series %d", w260) -> (resulting string=w258:string)  [unwired: 2 in, 1 out]
                  n100 = One Button Dialog(message=w258, button name ("OK")="stop") -> ()  [unwired: 1 out]
                }
                frame True {
                }
              }
            }
            frame #2 {
              w272 = 2 ("index")
              n101 = Reciprocal(x=w271) -> (1/x=w270:dbl)
              n102 = Array Size(array=w269) -> (size(s)=w273:i32)
              n103 = Divide(x=w270, y=w273) -> (x/y=w264:dbl)
              n104 = call "Power_spectrum.vi"("U"=w269, "Sampling frequency"=w270, "Block No"=1) -> ("Spectrum output array"=w267:dbl[])  [unwired: 1 in, 2 out]
              n105 = call <vilib>:"Std Deviation and Variance.vi"("X"=w269) -> ("variance"=w268:dbl)  [unwired: 1 in, 2 out]
              n106 = Array Subset(array=w267, index=w272) -> (w263:dbl[])  [unwired: 1 in]
              n107 = Divide(x=w267, y=w268) -> (x/y=w266:dbl[])
              n108 = Divide(x=w263, y=w268) -> (x/y=w262:dbl[])
              n109 = Array Size(array=w262) -> (size(s)=w276:i32)
              n110 = for {
                N: w276 -> [_]
                tunnel: [w281] -> w275 mode=indexing
                tunnel: w264 -> [w283]
                tunnel: w272 -> [w279]
                i -> [w284]
                n111 = Increment(x=w284) -> (x+1=w280:i32)
                n112 = Add(x=w280, y=w279) -> (x+y=w278:i32)
                n113 = Multiply(x=w278, y=w283) -> (x*y=w282:dbl)
                n114 = Reciprocal(x=w282) -> (1/x=w281:dbl)
              }
              n115 = Bundle(w275, w262) -> (w277:cluster{dbl[], dbl[]})  [unwired: 1 out]
              n116 = Add Array Elements(numeric array=w266) -> (sum=w265:dbl)
              n117 = Multiply(x=w265, y=w264) -> ()  [unwired: 1 out]
            }
          }
        }
        n118 = And Array Elements(Boolean array=w224) -> (logical AND=w223:bool)
      }
      frame "Do fitting?" {
        n119 = case shown="\"None\"" w287 {
          tunnel: ["Adjust Plot scales etc" "Poly fit to data"] -> _
          frame "None" {
          }
          frame "Linear", Default {
          }
        }
      }
      frame "Poly fit to data" {
        n120 = case shown="\"None\", Default" w303 {
          tunnel: [0 ("polynomial order") 1 ("polynomial order") 2 ("polynomial order") 3 ("polynomial order") 4 ("polynomial order")] -> w302
          frame "None", Default {
          }
          frame "Linear" {
          }
          frame "2nd Poly" {
          }
          frame "3rd Poly" {
          }
          frame "4th Poly" {
          }
        }
        n121 = for {
          tunnel: w301 -> [w325] mode=indexing
          tunnel: [w326] -> w300 mode=indexing
          tunnel: w302 -> [w324]
          tunnel: [w319] -> w297 mode=indexing
          tunnel: w296 -> [w318]
          tunnel: w295 -> [w317]
          w323 = 8  # Enhancement factor
          n122 = Unbundle(w325) -> ("Output"=w316:dbl[], "PercentageDifferenceArray"=w315:dbl[])
          n123 = call <vilib>:"General Polynomial Fit.vi"("Y"=w315, "polynomial order"=w324, "X"=w316) -> ("Polynomial Coefficients"=w313:dbl[])  [unwired: 9 in, 3 out]
          n124 = case shown="False" "Something about fit..!" {
            tunnel: [w329 w344] -> w320
            tunnel: [w340 w345] -> w319
            tunnel: w318 -> [w342 _]
            tunnel: w317 -> [w341 _]
            tunnel: w316 -> [w337 _]
            tunnel: w315 -> [w334 _]
            tunnel: w313 -> [_ w344]
            frame False {
              w336 = 0.99 ("Voltage")
              n125 = Build Array (concatenate)(nan ("Voltage"), w334) -> (w338:dbl[])
              n126 = Build Array (concatenate)(w336, w337) -> (w339:dbl[])
              n127 = call "Curve_Fit_ph.vi"("Values In"=w338, "No of points to fit (3)"=4, "Positions"=w339) -> ("Values Out"=w333:dbl[], "Polynomial Fit Coefficients"=w329:dbl[])  [unwired: 1 in]
              n128 = Index Array(array=w333, index=0) -> (element=w331:dbl)
              n129 = call "Number_2_string.vi"("precision"="2", "number"=w331) -> ("String"=w327:string)
              n130 = Format Into String(format string="When %s=%.2f ; %s=%s", w342, w336, w341, w327) -> (resulting string=w340:string)  [unwired: 2 in, 1 out]
            }
            frame True {
              n131 = for {
                shift-right: [w347] -> w345
                shift-left: "" -> [w348]
                tunnel: w344 -> [w351] mode=indexing
                i -> [w352]
                n132 = call "Number_2_string.vi"("number"=w351) -> ("String"=w349:string)  [unwired: 1 in]
                n133 = case shown="0, Default" w352 {
                  tunnel: [w353] -> w350
                  tunnel: w349 -> [w355]
                  frame 0, Default {
                    n134 = Concatenate Strings(w355, " ") -> (w353:string)
                  }
                }
                n135 = Concatenate Strings(w348, w350) -> (w347:string)
              }
            }
          }
          n136 = call "Enhance_No_of_points.vi"("Enhancement factor"=w323, "Input"=w316) -> ("Output"=w322:dbl[])  [unwired: 3 out]
          n137 = for {
            tunnel: w320 -> [w358]
            tunnel: w322 -> [w357] mode=indexing
            tunnel: [w356] -> w321 mode=indexing
            n138 = call "Polynomial_convert.vi"("Calib constants"=w358, "Voltage"=w357) -> ("Eng Values"=w356:dbl)  [unwired: 4 out]
          }
          n139 = Bundle("Output"=w322, w321) -> (w326:cluster{"Output":dbl[], dbl[]})  [unwired: 1 out]
        }
        n140 = Build Array (concatenate)(w299, w297) -> (w298:string[])
        n141 = Build Array (concatenate)(w301, w300) -> (w294:T7)
        n142 = local write "XY Graph"(w294) -> ()
      }
      frame "Add fitted line styles" {
        n143 = local read "No of Series"() -> (w359:i32)
        n144 = Array Subset(array=w362, index=w359) -> (w361:string[])  [unwired: 1 in]
        n145 = for {
          tunnel: w361 -> [w370] mode=indexing
          tunnel: u8 2 ("Plot.Plot Interpolation") -> [w376]
          tunnel: w359 -> [w372]
          i -> [w373]
          w378 = u32 0
          n146 = Concatenate Strings(w370, "  " ("string")) -> (w368:string)
          n147 = Add(x=w372, y=w373) -> (x+y=w371:i32)
          n148 = Quotient & Remainder(x=w373, y=4) -> (x-y*floor(x/y)=w374:i32)  [unwired: 1 out]
          n149 = property on="XY Graph" class="XYGraph (strict)"("Active Plot"=w371, "Plot.Plot Name"=w368, "Plot.Fill/Point Color"=w378, "Plot.Plot Color"=w378, "Plot.Point Style"=u8 0, "Plot.Line Style"=w374, "Plot.Plot Interpolation"=w376) -> ()  [unwired: 2 in, 2 out]
        }
      }
      frame "Adjust Plot scales etc" {
        w379 = u8[] [6, 1, 11, 2, 5, 13, 15, 10, 12, 14]  # pointStyles
        n150 = Greater Than 0?(x=w385) -> (x > 0?=w384:bool)
        n151 = Array Size(array=w387) -> (size(s)=w392:i32)
        n152 = local read "No of Series"() -> (w386:i32)
        n153 = property on="XY Graph" class="XYGraph (strict)"("Legend:Plots Shown"=w392) -> ()  [unwired: 2 in, 2 out]
        n154 = case shown="\"None\", Default" w382 {
          tunnel: ["Adjust plot scales2" "Show percentage change" ("t") "Set spectra axis" ("t") "Set spectra axis" ("t")] -> w381
          frame "None", Default {
          }
          frame "% change" {
          }
          frame "Spectrum" {
          }
          frame "Norm Spec" {
          }
        }
        n155 = Select(t=u8 2 ("Plot.Plot Interpolation"), s=w384, f=u8 0 ("Plot.Plot Interpolation")) -> (s? t:f=w388:u8)
        n156 = for {
          N: w386 -> [_]
          tunnel: w387 -> [w406] mode=indexing
          tunnel: w379 -> [w410]
          tunnel: w388 -> [w399]
          i -> [w409]
          w411 = u32 0
          n157 = String Length(string=w406) -> (length=w402:i32)
          n158 = Subtract(x=w402, y=2) -> (x-y=w400:i32)
          n159 = String Subset(string=w406, offset (0)=0, length (rest)=w400) -> (substring=w405:string)
          n160 = Concatenate Strings(w405, "  " ("string")) -> (w403:string)
          n161 = Index Array(array=w410, index=w409) -> (element=w408:u8)
          n162 = property on="XY Graph" class="XYGraph (strict)"("Active Plot"=w409, "Plot.Plot Name"=w403, "Plot.Fill/Point Color"=w411, "Plot.Plot Color"=w411, "Plot.Point Style"=w408, "Plot.Line Style"=u8 0, "Plot.Plot Interpolation"=w399) -> ()  [unwired: 2 in, 2 out]
        }
        "XY Graph" <- w380
      }
      frame "Adjust plot scales2" {
        n163 = property on="XY Graph" class="XYGraph (strict)"("X Scale.Name Label.Text"=w413, "Y Scale.Name Label.Text"=w412, "Cursor.Visible"=FALSE) -> ()  [unwired: 2 in, 2 out]
      }
      frame "Show percentage change" {
        n164 = Concatenate Strings(w424, " % Change" ("string")) -> (w427:string)
        n165 = property on="XY Graph" class="XYGraph (strict)"("X Scale.Name Label.Text"=w425, "Y Scale.Name Label.Text"=w427, "Cursor.Visible"=FALSE) -> ()  [unwired: 2 in, 2 out]
      }
      frame "Set spectra axis" {
        n166 = case shown="\"Spectrum\", Default" w432 {
          tunnel: [" Spectral Energy" ("string") " Normalised Spectral Energy" ("string")] -> w440
          frame "Spectrum", Default {
          }
          frame "Norm Spec" {
          }
        }
        n167 = Concatenate Strings(w437, w440) -> (w439:string)
        n168 = property on="XY Graph" class="XYGraph (strict)"("X Scale.Name Label.Text"="Wavelength [mm]", "Y Scale.Name Label.Text"=w439, "Cursor.Visible"=FALSE) -> ()  [unwired: 2 in, 2 out]
      }
      frame "Fill Second legend" {
        n169 = global read "Results_plotter_Global.vi" "Current Data Filenames"() -> (w450:string)
        n170 = call "Fast_string_Replace.vi"("Replace match with:"="_", "Input String"=w450, "regular expression"="[/]") -> ("Output String"=w454:string)  [unwired: 2 out]
        n171 = call "Fast_string_Replace.vi"("Replace match with:"="_", "Input String"=w454, "regular expression"="__") -> ("Output String"=w451:string)  [unwired: 2 out]
        n172 = call "Fast_string_Replace.vi"("Replace match with:"="", "Input String"=w451, "regular expression"=" ") -> ("Output String"=w449:string)  [unwired: 2 out]
        n173 = String Subset(string=w449, offset (0)=0, length (rest)=30 ("length (rest)")) -> (substring=w448:string)
        n174 = Build Path(base path=w461, name or relative path=w448) -> (appended path=w465:path)
      }
      frame "Calculate plot max and min values" {
        n175 = local read "plot error bars?"() -> (w468:bool)
        n176 = for {
          tunnel: w496 -> [w524] mode=indexing
          shift-right: [w521] -> w492
          shift-left: _ -> [w517]
          shift-right: [w520] -> w493
          shift-left: _ -> [w516]
          shift-right: [w519] -> w487
          shift-left: _ -> [w515]
          shift-right: [w518] -> w486
          shift-left: _ -> [w514]
          tunnel: w469 -> [w512]
          tunnel: w468 -> [w513]
          tunnel: w467 -> [w510]
          i -> [w511]
          n177 = Unbundle(w524) -> ("Output"=w523:dbl[], "PercentageDifferenceArray"=w522:dbl[])
          n178 = case shown="True" w513 {
            tunnel: w512 -> [_ w545]
            tunnel: w511 -> [_ w544]
            tunnel: [0.0 w540] -> w505
            frame False {
            }
            frame True {
              n179 = Index Array(array=w545, index=w544) -> (element=w543:cluster{string[]})
              n180 = Unbundle(w543) -> (w542:string[])
              n181 = Fract/Exp String To Number(string=w542) -> (number=w541:dbl[])  [unwired: 4 out]
              n182 = Array Max & Min(array=w541) -> (max value=w540:dbl)  [unwired: 3 out]
            }
          }
          n183 = Array Max & Min(array=w523) -> (max value=w503:dbl, min value=w501:dbl)  [unwired: 2 out]
          n184 = Array Max & Min(array=w522) -> (max value=w509:dbl, min value=w507:dbl)  [unwired: 2 out]
          n185 = case shown="True" w510 {
            tunnel: w509 -> [w531 w538]
            tunnel: [w530 w538] -> w508
            tunnel: w507 -> [w529 w537]
            tunnel: [w528 w537] -> w506
            tunnel: w505 -> [w527 w536]
            tunnel: [w526 w532] -> w504
            tunnel: w503 -> [w526 w535]
            tunnel: [w525 w533] -> w502
            tunnel: w501 -> [w525 w534]
            frame False {
              n186 = Subtract(x=w529, y=w527) -> (x-y=w528:dbl)
              n187 = Add(x=w531, y=w527) -> (x+y=w530:dbl)
            }
            frame True {
              n188 = Add(x=w535, y=w536) -> (x+y=w532:dbl)
              n189 = Subtract(x=w534, y=w536) -> (x-y=w533:dbl)
            }
          }
          n190 = case shown="1, Default" w511 {
            tunnel: [w549 w563] -> w521
            tunnel: w504 -> [w549 w562]
            tunnel: w502 -> [w548 w559]
            tunnel: [w548 w558] -> w520
            tunnel: [w547 w551] -> w519
            tunnel: w508 -> [w547 w554]
            tunnel: [w546 w550] -> w518
            tunnel: w506 -> [w546 w552]
            tunnel: w517 -> [_ w564]
            tunnel: w516 -> [_ w561]
            tunnel: w515 -> [_ w555]
            tunnel: w514 -> [_ w553]
            frame 0 {
            }
            frame 1, Default {
              n191 = Greater?(x=w555, y=w554) -> (0:w556:bool)
              n192 = Greater?(x=w564, y=w562) -> (0:w565:bool)
              n193 = Less?(x=w553, y=w552) -> (x < y?=w557:bool)
              n194 = Less?(x=w561, y=w559) -> (x < y?=w560:bool)
              n195 = Select(t=w555, s=w556, f=w554) -> (s? t:f=w551:dbl)
              n196 = Select(t=w553, s=w557, f=w552) -> (s? t:f=w550:dbl)
              n197 = Select(t=w564, s=w565, f=w562) -> (s? t:f=w563:dbl)
              n198 = Select(t=w561, s=w560, f=w559) -> (s? t:f=w558:dbl)
            }
          }
        }
        n199 = Subtract(x=w492, y=w493) -> (x-y=w494:dbl)
        n200 = Subtract(x=w487, y=w486) -> (x-y=w489:dbl)
        n201 = Multiply(x=w494, y=0.1) -> (x*y=w491:dbl)
        n202 = Multiply(x=w489, y=0.1) -> (x*y=w490:dbl)
        n203 = Add(x=w492, y=w491) -> (x+y=w479:dbl)
        n204 = Subtract(x=w493, y=w491) -> (x-y=w476:dbl)
        n205 = Add(x=w487, y=w490) -> (x+y=w472:dbl)
        n206 = Subtract(x=w486, y=w490) -> (x-y=w481:dbl)
        n207 = Select(t=w479, s="Xmax", f="Xmax Val") -> (s? t:f=w477:dbl)
        n208 = Select(t=w476, s="Xmin", f="Xmin Val") -> (s? t:f=w484:dbl)
        n209 = Select(t=w472, s="Ymax", f="Ymax Val") -> (s? t:f=w470:dbl)
        n210 = Select(t=w481, s="Ymin", f="Ymin Val") -> (s? t:f=w485:dbl)
        n211 = property on="XY Graph" class="XYGraph (strict)"("X Scale.Range:Maximum"=w477, "X Scale.Range:Minimum"=w484, "Y Scale.Range:Maximum"=w470, "Y Scale.Range:Minimum"=w485) -> ()  [unwired: 2 in, 2 out]
      }
      frame "Sort out plot title" {
        n212 = local read "Summarise"() -> (w579:u16)
        n213 = case shown="1, Default" "Plot Title" {
          selector: "Plot Title" -> [_ w596]
          tunnel: [w595 w602] -> w574
          tunnel: "Plot Title" -> [w595 w601]
          tunnel: w575 -> [_ w605]
          tunnel: w579 -> [_ w599]
          frame 0 {
          }
          frame 1, Default {
            n214 = Decrement(x=w596) -> (x-1=w604:u16)
            n215 = Add(x=w599, y=u16 2) -> (x+y=w598:u16)
            n216 = Index Array(array=w605, index (row)=w604, index (col)=w598) -> (element=w608:string)
            n217 = Empty String/Path?(string/path=w601) -> (empty?=w603:bool)
            n218 = call "Fast_string_Replace.vi"("Replace match with:"="~ ", "Input String"=w608, "regular expression"=":") -> ("Output String"=w607:string)  [unwired: 2 out]
            n219 = call <vilib>:"Trim Whitespace.vi"("string"=w607) -> ("trimmed string"=w606:string)  [unwired: 1 in]
            n220 = call "Fast_string_Replace.vi"("Replace match with:"="~", "Input String"=w606, "regular expression"="_") -> ("Output String"=w597:string)  [unwired: 2 out]
            n221 = case shown="False" w603 {
              tunnel: [w614 w617] -> w602
              tunnel: w597 -> [w616 w617]
              tunnel: w601 -> [w615 _]
              frame False {
                n222 = Concatenate Strings(w615, " " ("string"), w616) -> (w614:string)
              }
              frame True {
              }
            }
          }
        }
        n223 = case shown="True" "Show Labels?" {
          tunnel: w575 -> [w590 _]
          tunnel: w574 -> [w593 w594]
          tunnel: [w591 w594] -> w573
          frame False {
            n224 = local read "Added labels"() -> (w592:i32[])
            n225 = Concatenate Strings(w593, "         " ("string")) -> (w589:string)
            n226 = call "DistillTitle.vi"("Plot Summary in"=w590, "Indices to include in Page Title"=w592, "String in"=w589) -> ("String out"=w591:string)  [unwired: 7 in, 1 out]
          }
          frame True {
          }
        }
        "Final Title" <- w573
        n227 = Current VI's Path() -> (path=w571:path)
        n228 = call "Running_as_top_level.vi"("Vi path name"=w571) -> ("Top Level"=w569:bool)  [unwired: 1 out]
        n229 = case shown="True" w569 {
          tunnel: [w583 w586] -> w568
          tunnel: w567 -> [w583 _]
          tunnel: ["Get Filename" ("t") "Create plot directory"] -> w566
          frame False {
          }
          frame True {
            n230 = local read "Path"() -> (w585:path)
            n231 = Strip Path(path=w585) -> (name=w584:string)  [unwired: 1 out]
            n232 = Build Path(base path=w585, name or relative path=w584) -> (appended path=w586:path)
          }
        }
      }
      frame "Get Filename" {
        n233 = local read "Final Title"() -> (w621:string)
        n234 = case shown="\"% change\"" w623 {
          tunnel: ["" "Per_" "Spec_" "N_Spec_"] -> w622
          frame "None" {
          }
          frame "% change" {
          }
          frame "Spectrum" {
          }
          frame "Norm Spec" {
          }
        }
        n235 = Concatenate Strings(w622, w621) -> (w618:string)
        n236 = String Length(string=w621) -> (length=w620:i32)
        n237 = case shown="1, Default" w620 {
          tunnel: [w638 w639] -> w619
          tunnel: w618 -> [w638 w641]
          frame 0 {
          }
          frame 1, Default {
            n238 = Concatenate Strings(w641, "_") -> (w639:string)
          }
        }
        n239 = call "Auto_filename.vi"("Filename Max length"="Filename Max length", "Prefix"=w619) -> ("Filename"=w625:string)
        n240 = Build Path(base path=w632, name or relative path=w625) -> (appended path=w629:path)
        n241 = File/Directory Info(path=w629) -> (error out=w630:errorcluster)  [unwired: 1 in, 6 out]
        n242 = Build Path(base path=w629, name or relative path=w625) -> (appended path=w636:path)
        n243 = Unbundle By Name(w630) -> ("status"=w628:bool)
        n244 = Select(t="Create plot directory", s=w628, f="Find a unique name") -> (s? t:f=w635:string)
      }
      frame "Find a unique name" {
        n245 = call "FindUniqueName.vi"("Max Length"=27, "PathIn"=w648) -> ("UniquedPath"=w647:path)  [unwired: 9 in]
      }
      frame "Create plot directory" {
        n246 = Strip Path(path=w656) -> (stripped path=→"Path":path)  [unwired: 1 out]
        n247 = case shown="True" "Call GNUPLOT" {
          tunnel: [w665 w667] -> w661
          tunnel: w656 -> [w665 w666]
          frame False {
          }
          frame True {
            n248 = call "Create_directory_path.vi"("Path name"=w666) -> ("Path name Out"=w667:path)  [unwired: 1 in, 1 out]
          }
        }
        n249 = Select(t="Save data analysis file", s="Save data analysis file", f="Save .dat file") -> (s? t:f=w659:string)
      }
      frame "Save data analysis file" {
        n250 = stacked-sequence {
          seq-local: [w679 _ _] -> [_ _ w723]
          seq-local: [_ w695 _] -> [_ _ w721]
          tunnel: w677 -> [_ _ w734]
          tunnel: [_ _ TRUE ("Top Level")] -> w676
          tunnel: [_ _ "Save .dat file"] -> w675
          tunnel: w674 -> [w682 w697 _]
          tunnel: w673 -> [_ _ _]
          tunnel: w672 -> [_ _ _]
          tunnel: w668 -> [_ w698 _]
          tunnel: w670 -> [w686 _ _]
          tunnel: w669 -> [w685 _ _]
          frame #0 {
            n251 = case shown="\"Norm Spec\"" w686 {
              tunnel: w685 -> [w689 w693]
              tunnel: [w688 w692] -> w684
              tunnel: ["Wavelength::[mm]" "Wavelength::[mm]"] -> w683
              frame "Spectrum", Default {
                n252 = Concatenate Strings(w689, ":Spectral:Energy") -> (w688:string)
              }
              frame "Norm Spec" {
                n253 = Concatenate Strings(w693, ":Normalised Spectral:Energy") -> (w692:string)
              }
            }
            n254 = Index Array(array=w682, index (col)=0 ("disabled index (col)")) -> (element=w680:string[])  [unwired: 1 in]
            n255 = Build Array (concatenate)(w683, w684, w680) -> (w679:string[])
          }
          frame #1 {
            n256 = for {
              tunnel: w698 -> [w709] mode=indexing
              tunnel: w697 -> [w706]
              shift-right: [w700] -> w695
              shift-left: string[][] [] -> [w699]
              i -> [w704]
              n257 = Unbundle(w709) -> ("Output"=w708:dbl[], "PercentageDifferenceArray"=w707:dbl[])
              n258 = Add(x=3 ("disabled index (col)"), y=w704) -> (x+y=w703:i32)
              n259 = Index Array(array=w706, index (col)=w703) -> (element=w702:string[])  [unwired: 1 in]
              n260 = for {
                tunnel: w708 -> [w715] mode=indexing
                tunnel: w707 -> [w714] mode=indexing
                tunnel: w702 -> [w711]
                tunnel: [w710] -> w701 mode=indexing
                n261 = call "Number_2_string.vi"("number"=w715) -> ("String"=w713:string)  [unwired: 1 in]
                n262 = call "Number_2_string.vi"("number"=w714) -> ("String"=w712:string)  [unwired: 1 in]
                n263 = Build Array (concatenate)(w713, w712, w711) -> (w710:string[])
              }
              n264 = Build Array (concatenate)(w699, w701) -> (w700:string[][])
            }
          }
          frame #2 {
            w730 = FALSE  # Append last row only
            w729 = FALSE  # exists?
            n265 = Strip Path(path=w734) -> (stripped path=w735:path, name=w737:string)
            n266 = Array Size(array=w721) -> (size(s)=w720:i32[])
            n267 = Concatenate Strings(w737, ".xls" ("string")) -> (w736:string)
            n268 = Index Array(array=w720, index=0) -> (element=w718:i32)
            n269 = Build Path(base path=w735, name or relative path=w736) -> (appended path=w724:path)
            n270 = Initialize Array("", w718) -> (w717:string[])
            n271 = Build Array (concatenate)(w717, w721) -> (w722:string[][])
            n272 = Initialize Array("", 10 ("Dimension Size")) -> (w728:string[])
            n273 = call "Asterisk_header.vi"("Channel names"=w728) -> ("Header string"=w725:string)
            n274 = call "Write_Ch_data_file.vi"("Append last row only"=w730, "Header string"=w725, "exists?"=w729, "Channel Values"=w722, "Channel names"=w723, "Filename"=w724) -> ()  [unwired: 2 in, 4 out]
          }
        }
      }
      frame "Save .dat file" {
        n275 = stacked-sequence {
          seq-local: [w752 _ _ _ _] -> [_ _ _ _ w872]
          seq-local: [_ w778 _ _ _] -> [_ _ _ _ w873]
          seq-local: [_ _ _ w811 _] -> [_ _ _ _ w874]
          seq-local: [_ _ w795 _ _] -> [_ _ _ w809 _]
          seq-local: [_ _ w787 _ _] -> [_ _ _ w806 _]
          seq-local: [_ _ w789 _ _] -> [_ _ _ w805 _]
          tunnel: w750 -> [_ _ _ _ w877]
          tunnel: [_ _ _ _ TRUE ("Top Level")] -> w749
          tunnel: [_ _ _ _ "Gnuplot script Start"] -> w748
          tunnel: w747 -> [w757 _ _ _ _]
          tunnel: w746 -> [_ w781 _ _ _]
          tunnel: w745 -> [_ w777 _ _ _]
          tunnel: w744 -> [_ _ _ w813 _]
          tunnel: w743 -> [_ _ _ w810 _]
          tunnel: w742 -> [_ w775 _ _ _]
          tunnel: [_ _ _ w808 _] -> w741
          tunnel: w740 -> [_ _ w793 _ _]
          tunnel: w739 -> [_ _ _ w807 _]
          tunnel: w738 -> [_ _ w790 _ _]
          frame #0 {
            n276 = Array Subset(array=w757, length (col)=3 ("length")) -> (w755:string[][])  [unwired: 3 in]
            n277 = Build Array("Column Name", "Numeric Tolerance", "Range of Values") -> (w761:string[])
            n278 = Build Array (concatenate)(w761, w755) -> (w753:string[][])
            n279 = for {
              shift-right: [w765] -> w752
              shift-left: "" -> [w762]
              tunnel: w753 -> [w766] mode=indexing
              n280 = for {
                shift-right: [w767] -> w764
                shift-left: w762 -> [w774]
                tunnel: w766 -> [w768] mode=indexing
                i -> [w773]
                n281 = Equal To 0?(x=w773) -> (x = 0?=w772:bool)
                n282 = Select(t="#", s=w772, f="\t") -> (s? t:f=w769:string)
                n283 = Concatenate Strings(w774, w769, w768) -> (w767:string)
              }
              n284 = Concatenate Strings(w764, "\n") -> (w765:string)
            }
          }
          frame #1 {
            w779 = "\n"
            n285 = case shown="\"% change\"" w775 {
              tunnel: w777 -> [w783 w785]
              tunnel: [w783 w784] -> w776
              frame "None", Default {
              }
              frame "% change" {
                n286 = Concatenate Strings(w785, " %" ("string")) -> (w784:string)
              }
            }
            n287 = Concatenate Strings(w779, w779, "#" ("string"), w781, "\t", w776, w779, w779) -> (w778:string)
          }
          frame #2 {
            n288 = global read "Results_plotter_Global.vi" "Precision"() -> (w792:string[])
            n289 = global read "Results_plotter_Global.vi" "Absisca"() -> (w791:i32)
            n290 = case shown="True" "Offset?" {
              tunnel: [0.0 w803] -> w796
              frame False {
              }
              frame True {
                n291 = property on="XY Graph" class="XYGraph (strict)"() -> ("Y Scale.Range:Maximum"=w802:dbl, "Y Scale.Range:Minimum"=w804:dbl)  [unwired: 2 in, 2 out]
                n292 = Subtract(x=w802, y=w804) -> (x-y=w803:dbl)
              }
            }
            "Profile offset" <- w796
            n293 = Index Array(array=w792, index=w791) -> (element=w788:string)
            n294 = case shown="False" w790 {
              tunnel: ["" w800] -> w789
              tunnel: w788 -> [w797 w800]
              tunnel: [w797 ""] -> w787
              frame False {
              }
              frame True {
              }
            }
            n295 = Multiply(x=w796, y=w793) -> (x*y=w795:dbl)
          }
          frame #3 {
            n296 = for {
              tunnel: w813 -> [w840] mode=indexing
              shift-right: [w839] -> w811
              shift-left: "" -> [w830]
              tunnel: w810 -> [w828] mode=indexing
              tunnel: w809 -> [w825]
              tunnel: [w831] -> w808 mode=indexing
              tunnel: w807 -> [w818] mode=indexing
              tunnel: w806 -> [w815]
              tunnel: w805 -> [w814]
              i -> [w835]
              w838 = "\n"
              n297 = Multiply(x=w825, y=w835) -> (x*y=w820:dbl)
              n298 = Unbundle(w840) -> ("Output"=w833:dbl[], "PercentageDifferenceArray"=w834:dbl[])
              n299 = Negate(x=w820) -> (-x=w819:dbl)
              n300 = call "Number_2_string.vi"("number"=w819) -> ("String"=w827:string)  [unwired: 1 in]
              n301 = Format Into String(format string="\\t%s\\tPlot offset", w827) -> (resulting string=w823:string)  [unwired: 2 in, 1 out]
              n302 = Equal To 0?(x=w820) -> (x = 0?=w824:bool)
              n303 = Select(t="", s=w824, f=w823) -> (s? t:f=w821:string)
              n304 = Unbundle(w818) -> (w817:string[])
              n305 = for {
                tunnel: w833 -> [w859] mode=indexing
                shift-right: [w848] -> w837
                shift-left: "" -> [w849]
                tunnel: w834 -> [w856] mode=indexing
                tunnel: w820 -> [w855]
                tunnel: [w854] -> w832 mode=indexing
                tunnel: w817 -> [w851]
                shift-right: [w847] -> _
                shift-left: string[] [] -> [w846]
                tunnel: w815 -> [w843]
                tunnel: w814 -> [w842]
                i -> [w852]
                w853 = "\t"
                n306 = Subtract(x=w856, y=w855) -> (x-y=w854:dbl)
                n307 = call "Number_2_string.vi"("precision"=w843, "number"=w859) -> ("String"=w858:string)
                n308 = call "Number_2_string.vi"("precision"=w842, "number"=w854) -> ("String"=w857:string)
                n309 = Index Array(array=w851, index=w852) -> (element=w850:string)
                n310 = Concatenate Strings(w858, w853, w857, w853, w850, "\n") -> (w845:string)
                n311 = Search 1D Array(1D array=w846, element=w845) -> (index of element=w844:i32)  [unwired: 1 in]
                n312 = case shown="-1" w844 {
                  tunnel: w849 -> [w861 w866]
                  tunnel: [w861 w865] -> w848
                  tunnel: w845 -> [_ w862]
                  tunnel: w846 -> [w860 w864]
                  tunnel: [w860 w863] -> w847
                  frame 0, Default {
                  }
                  frame -1 {
                    n313 = Concatenate Strings(w866, w862) -> (w865:string)
                    n314 = Build Array (concatenate)(w864, w862) -> (w863:string[])
                  }
                }
              }
              n315 = Bundle("Output"=w833, w832) -> (w831:cluster{"Output":dbl[], dbl[]})  [unwired: 1 out]
              n316 = Concatenate Strings(w830, "#", w828, w821, w838, w837, w838, w838) -> (w839:string)
            }
          }
          frame #4 {
            w869 = FALSE  # advisory dialog? (display:T)
            w870 = FALSE  # append to file? (new file:F)
            n317 = Strip Path(path=w877) -> (stripped path=w878:path, name=w880:string)
            n318 = Concatenate Strings(w872, w873, w874) -> (w871:string)
            n319 = Concatenate Strings(w880, ".dat" ("string")) -> (w879:string)
            n320 = Build Path(base path=w878, name or relative path=w879) -> (appended path=w868:path)
            n321 = call "Write_Characters_To_File.vi"("file path (dialog if empty)"=w868, "advisory dialog? (display:T)"=w869, "character string"=w871, "append to file? (new file:F)"=w870) -> ()  [unwired: 1 in, 4 out]
          }
        }
      }
      frame "Gnuplot script Start" {
        n322 = case shown="\"None\", Default" w901 {
          tunnel: w900 -> [w918 w921 w925 w929]
          tunnel: [w918 w920 w924 w928] -> w888
          tunnel: [w917 w919 "Wavelength [mm]" ("X Axis Name") "Wavelength [mm]" ("X Axis Name")] -> w887
          tunnel: w899 -> [w917 w919 _ _]
          frame "None", Default {
          }
          frame "% change" {
            n323 = Concatenate Strings(w921, " % change" ("string")) -> (w920:string)
          }
          frame "Spectrum" {
            n324 = Concatenate Strings(w925, " Spectral energy" ("string")) -> (w924:string)
          }
          frame "Norm Spec" {
            n325 = Concatenate Strings(w929, " Normalised Spectral Energy" ("string")) -> (w928:string)
          }
        }
        n326 = local read "Final Title"() -> (w889:string)
        n327 = case shown="\"Linear\", Default" w893 {
          tunnel: [w908 w910 "Calculate fit parameters"] -> w892
          tunnel: "Edit Legend names" -> [w908 w910 _]
          tunnel: [w907 w909 "set parametric\nset samples 1000\n"] -> w881
          tunnel: "" -> [w907 w909 _]
          frame "None" {
          }
          frame "Spline" {
          }
          frame "Linear", Default {
          }
        }
        n328 = call "setTerm.vi"() -> ("String out"=w886:string)  [unwired: 10 in, 1 out]
        n329 = call "TypesetInsideMathmode.vi"("DirtyString"=w887) -> ("Mathmode String"=w883:string)  [unwired: 9 in, 1 out]
        n330 = call "TypesetInsideMathmode.vi"("DirtyString"=w888) -> ("Mathmode String"=w882:string)  [unwired: 9 in, 1 out]
        n331 = call "TypesetInsideMathmode.vi"("DirtyString"=w889) -> ("Mathmode String"=w885:string)  [unwired: 9 in, 1 out]
        n332 = local read "Time format?"() -> (w894:bool)
        n333 = call "setTitle.vi"("Title"=w885, "String in"=w886) -> ("String out"=w884:string)  [unwired: 8 in, 1 out]
        n334 = Format Into String(format string="set xlabel '%s'\nset ylabel '%s'\nset size %s,%s\n%s", initial string=w884, w883, w882, "Graph width", "Graph Height", w881) -> (resulting string=w896:string)  [unwired: 1 in, 1 out]
        n335 = case shown="True" w894 {
          tunnel: w896 -> [w913 w915]
          tunnel: [w913 w914] -> w895
          frame False {
          }
          frame True {
            n336 = Concatenate Strings(w915, "\nset xdata time\nset timefmt \"%s\"\nset format  x \"%d %H:%M\"\n") -> (w914:string)
          }
        }
      }
      frame "Calculate fit parameters" {
        # "k=1;    # label 1\nlab=\"23 mA\";\neval( sprintf (\"set label %d %s\", k, lab))"
        n337 = Strip Path(path=w944) -> (name=w943:string)  [unwired: 1 out]
        n338 = Select(t="2:1", s=w932, f="1:2") -> (s? t:f=w933:string)
        n339 = for {
          tunnel: w946 -> [w961]
          tunnel: w943 -> [w959]
          shift-right: [w957] -> w939
          shift-left: w942 -> [w958]
          tunnel: "Auto Zp" -> [w956]
          tunnel: "Fixed Zp" -> [w955]
          tunnel: w933 -> [w954]
          tunnel: w932 -> [w953]
          tunnel: w931 -> [w952] mode=indexing
          i -> [w960]
          n340 = Unbundle(w952) -> ("Output"=w950:dbl[], "PercentageDifferenceArray"=w948:dbl[])
          n341 = case shown="False" w953 {
            tunnel: [w963 w965] -> w951
            tunnel: w950 -> [w963 w964]
            tunnel: [w962 w964] -> w949
            tunnel: w948 -> [w962 w965]
            frame False {
            }
            frame True {
            }
          }
          n342 = case shown="\"Gauss Vert with 2 sig\"" w961 {
            tunnel: w960 -> [w974 w994 w1010 w1029 w1053 w1057 w1063 w1069 _]
            tunnel: w959 -> [w976 w995 w1004 w1034 w1054 w1058 w1064 w1070 _]
            tunnel: w958 -> [w984 w999 w1019 w1044 w1052 w1060 w1066 w1072 w1074]
            tunnel: [w983 w998 w1018 w1043 w1051 w1059 w1065 w1071 w1074] -> w957
            tunnel: w956 -> [_ _ w1009 w1033 _ _ _ _ _]
            tunnel: w955 -> [_ _ w1006 w1030 _ _ _ _ _]
            tunnel: w954 -> [w966 w986 w1003 w1025 w1050 w1056 w1062 w1068 _]
            tunnel: w951 -> [w967 w987 w1002 w1027 _ _ _ _ _]
            tunnel: w949 -> [w968 w988 w1001 w1026 _ _ _ _ _]
            frame "Gauss Lat" {
              w971 = 0.01  # A value of zero make gnuplot stop working
              n343 = Array Max & Min(array=w968) -> (max value=w978:dbl, max index (indices)=w975:i32)  [unwired: 2 out]
              n344 = Array Max & Min(array=w967) -> (max value=w982:dbl, min value=w981:dbl)  [unwired: 2 out]
              n345 = Index Array(array=w967, index=w975) -> (element=w970:dbl)
              n346 = Subtract(x=w982, y=w981) -> (x-y=w980:dbl)
              n347 = Divide(x=w980, y=6.0) -> (x/y=w977:dbl)
              n348 = Absolute Value(x=w970) -> (abs(x)=w972:dbl)
              n349 = Greater?(x=w972, y=w971) -> (0:w973:bool)
              n350 = Select(t=w970, s=w973, f=w971) -> (s? t:f=w969:dbl)
              n351 = Format Into String(format string="\nf%d(t) = cmax%d*exp(-((t-offset%d)**2)/(2*sig%d**2))\ncmax%d = %.2f; sig%d = %.2f; offset%d = %.2f           # initial guess for cmax and sig and offset\nfit f%d(t) \"%s.dat\" index %d using %s via cmax%d, sig%d, offset%d #this is a gaussian fit\n", initial string=w984, w974, w974, w974, w974, w974, w978, w974, w977, w974, w969, w974, w976, w974, w966, w974, w974, w974) -> (resulting string=w983:string)  [unwired: 1 in, 1 out]
            }
            frame "Guass glc" {
              w991 = 0.01 ("y")
              n352 = Array Max & Min(array=w988) -> (max value=w997:dbl, max index (indices)=w996:i32)  [unwired: 2 out]
              n353 = Index Array(array=w987, index=w996) -> (element=w990:dbl)
              n354 = Absolute Value(x=w990) -> (abs(x)=w992:dbl)
              n355 = Greater?(x=w992, y=w991) -> (0:w993:bool)
              n356 = Select(t=w990, s=w993, f=w991) -> (s? t:f=w989:dbl)
              n357 = Format Into String(format string="\nf%d(t) = cmax%d*((t/xmax%d)**(-(1+m%d)*q%d)*exp(((1+m%d)/2)*(1-(t/xmax%d)**(-2*q%d))))\ncmax%d = %.2f; xmax%d = %.2f; m%d = 1;  q%d = 0.73         # initial guess for cmax and xmax q and m\nfit f%d(t) \"%s.dat\" index %d using %s via cmax%d, xmax%d, m%d, q%d  #this is a gaussian fit\n", initial string=w999, w994, w994, w994, w994, w994, w994, w994, w994, w994, w997, w994, w989, w994, w994, w994, w995, w994, w986, w994, w994, w994, w994) -> (resulting string=w998:string)  [unwired: 1 in, 1 out]
            }
            frame "Gauss vert" {
              (unwired) "f1(x) = cmax1*exp(-((x-offset1)**2)/(2*sig1**2))"
              n358 = Array Max & Min(array=w1001) -> (max value=w1013:dbl, max index (indices)=w1011:i32)  [unwired: 2 out]
              n359 = Array Max & Min(array=w1002) -> (max value=w1017:dbl, min value=w1016:dbl)  [unwired: 2 out]
              n360 = Index Array(array=w1002, index=w1011) -> (element=w1008:dbl)
              n361 = Subtract(x=w1017, y=w1016) -> (x-y=w1015:dbl)
              n362 = Divide(x=w1015, y=6.0) -> (x/y=w1012:dbl)
              n363 = case shown="False" w1009 {
                tunnel: [w1022 w1024] -> w1007
                tunnel: w1008 -> [_ w1024]
                tunnel: w1006 -> [w1022 _]
                tunnel: [w1021 ""] -> w1005
                frame False {
                  w1021 = " #"  # #
                }
                frame True {
                }
              }
              n364 = Format Into String(format string="\nf%d(t) = cmax%d*(exp(-((t-Zp%d)**2)/(2*sigZ%d**2))+exp(-((t+Zp%d)**2)/(2*sigZ%d**2)))\ncmax%d = %.2f; sigZ%d = %.2f; Zp%d = %.2f           # initial guess for cmax and sig and offset\nfit f%d(t) \"%s.dat\" index %d using %s via cmax%d, sigZ%d%s, Zp%d #this is a gaussian fit\n", initial string=w1019, w1010, w1010, w1010, w1010, w1010, w1010, w1010, w1013, w1010, w1012, w1010, w1007, w1010, w1004, w1010, w1003, w1010, w1010, w1005, w1010) -> (resulting string=w1018:string)  [unwired: 1 in, 1 out]
            }
            frame "Gauss Vert with 2 sig" {
              n365 = Array Max & Min(array=w1026) -> (max value=w1036:dbl, max index (indices)=w1038:i32)  [unwired: 2 out]
              n366 = Array Max & Min(array=w1027) -> (max value=w1042:dbl, min value=w1041:dbl)  [unwired: 2 out]
              n367 = Index Array(array=w1027, index=w1038) -> (element=w1032:dbl)
              n368 = Subtract(x=w1042, y=w1041) -> (x-y=w1040:dbl)
              n369 = Divide(x=w1040, y=6.0) -> (x/y=w1035:dbl)
              n370 = call "Vert_Spread_2_Sig.vi"("Index"=w1029) -> ("resulting string"=w1037:string)
              n371 = case shown="False" w1033 {
                tunnel: [w1047 w1049] -> w1031
                tunnel: w1030 -> [w1047 _]
                tunnel: [w1046 ""] -> w1028
                tunnel: w1032 -> [_ w1049]
                frame False {
                  w1046 = " #"  # #
                }
                frame True {
                }
              }
              n372 = Format Into String(format string="\nf%d(t) = %s\ncmax%d = %.2f; sigZ_low%d = %.2f; sigZ_up%d = %.2f; Zp%d = %.2f           # initial guess for cmax and sig and offset\nfit f%d(t) \"%s.dat\" index %d using %s via cmax%d, sigZ_low%d, sigZ_up%d%s, Zp%d #this is a gaussian fit\n", initial string=w1044, w1029, w1037, w1029, w1036, w1029, w1035, w1029, w1035, w1029, w1031, w1029, w1034, w1029, w1025, w1029, w1029, w1029, w1028, w1029) -> (resulting string=w1043:string)  [unwired: 1 in, 1 out]
            }
            frame "2nd Poly" {
              n373 = Format Into String(format string="\nf%d(t) = c%d*t**2 + b%d*t + a%d\n#a%d = 40; b%d = 300; c%d = 1           # initial guess for cmax and sig and offset\nfit f%d(t) \"%s.dat\" index %d using %s via a%d, b%d, c%d #this is a 2nd order poly fit\n", initial string=w1052, w1053, w1053, w1053, w1053, w1053, w1053, w1053, w1053, w1054, w1053, w1050, w1053, w1053, w1053) -> (resulting string=w1051:string)  [unwired: 1 in, 1 out]
            }
            frame "3rd Poly" {
              n374 = Format Into String(format string="\nf%d(t) = d%d*t**3 +c%d*t**2 + b%d*t + a%d\n#a%d = 40; b%d = 300; c%d = 1; d%d = 1         # initial guess for cmax and sig and offset\nfit f%d(t) \"%s.dat\" index %d using %s via a%d, b%d, c%d, d%d #this is a 3rd order poly fit\n", initial string=w1060, w1057, w1057, w1057, w1057, w1057, w1057, w1057, w1057, w1057, w1057, w1058, w1057, w1056, w1057, w1057, w1057, w1057) -> (resulting string=w1059:string)  [unwired: 1 in, 1 out]
            }
            frame "4th Poly" {
              n375 = Format Into String(format string="\nf%d(t) = e%d*t**4 + d%d*t**3 +c%d*t**2 + b%d*t + a%d\n#a%d = 40; b%d = 300; c%d = 1; d%d = 1  e%d = 1       # initial guess for cmax and sig and offset\nfit f%d(t) \"%s.dat\" index %d using %s via a%d, b%d, c%d, d%d, e%d #this is a 3rd order poly fit\n", initial string=w1066, w1063, w1063, w1063, w1063, w1063, w1063, w1063, w1063, w1063, w1063, w1063, w1063, w1064, w1063, w1062, w1063, w1063, w1063, w1063, w1063) -> (resulting string=w1065:string)  [unwired: 1 in, 1 out]
            }
            frame "Linear" {
              n376 = Format Into String(format string="\nf%d(t) = b%d*t + c%d\n#a%d = 40; b%d = 300; c%d = 1           # initial guess for cmax and sig and offset\nfit f%d(t) \"%s.dat\" index %d using %s via b%d, c%d #this is a Linear fit\n", initial string=w1072, w1069, w1069, w1069, w1069, w1069, w1069, w1069, w1070, w1069, w1068, w1069, w1069) -> (resulting string=w1071:string)  [unwired: 1 in, 1 out]
            }
            frame "Spline", Default {
            }
          }
        }
        n377 = Concatenate Strings(w939, "save variables 'Coeff.txt'\n") -> (w940:string)
      }
      frame "Edit Legend names" {
        n378 = local read "Profile offset"() -> (w1083:dbl)
        n379 = for {
          tunnel: w1093 -> [w1108] mode=indexing
          tunnel: [w1107] -> w1092 mode=indexing
          tunnel: [w1106] -> w1088
          i -> [w1106]
          n380 = String Length(string=w1108) -> (length=w1111:i32)
          n381 = Subtract(x=w1111, y=2) -> (x-y=w1109:i32)
          n382 = String Subset(string=w1108, length (rest)=w1109) -> (substring=w1096:string)  [unwired: 1 out]
          n383 = Match Pattern(string=w1096, regular expression="=") -> (before substring=w1095:string, match substring=w1094:string, after substring=w1100:string)  [unwired: 2 out]
          n384 = call "Match_Pat_Case_In.vi"("String to match"="legend", "String"=w1095) -> ("offset past match"=w1103:i32)  [unwired: 1 in, 3 out]
          n385 = call "Fast_string_Replace.vi"("Replace match with:"=" ", "Input String"=w1100, "regular expression"="_") -> ("Output String"=w1097:string)  [unwired: 2 out]
          n386 = Greater Than 0?(x=w1103) -> (x > 0?=w1099:bool)
          n387 = case shown="False" w1099 {
            tunnel: [w1112 w1116] -> w1098
            tunnel: w1097 -> [w1113 w1116]
            tunnel: w1095 -> [w1115 _]
            tunnel: w1094 -> [w1114 _]
            frame False {
              n388 = Concatenate Strings(w1115, w1114, w1113) -> (w1112:string)
            }
            frame True {
            }
          }
          n389 = call "Text_for_latex.vi"("Input String"=w1098) -> ("Output String"=w1107:string)
        }
        n390 = Multiply(x=w1085, y=w1083) -> (x*y=w1087:dbl)
        n391 = Decrement(x=w1085) -> (x-1=w1084:dbl)
        n392 = Multiply(x=w1087, y=w1088) -> (x*y=w1082:dbl)
        n393 = Multiply(x=w1083, y=w1084) -> (x*y=w1081:dbl)
        n394 = Add(x=w1081, y=w1082) -> (x+y=→"Extra range":dbl)
        n395 = Equal To 0?(x="Legend Position") -> (x = 0?=w1078:bool)
        n396 = Select(t="Auto Legend Position", s=w1078, f="Specified Legend Position") -> (s? t:f=w1076:string)
      }
      frame "Auto Legend Position" {
        w1119 = T9 {"Appearance"={"layout"="horizontal", "text-sample order"="", "key order"="", "surroundingBox"=""}, "Alignment"={"Horizontal"="center", "Vertical"="bottom"}, "Location"="", "\"At\" location"={"XcoordSys"="", "YcoordSys"="", "Xvalue"=0.0, "Yvalue"=0.0}}  # LegendProperties
        w1117 = "at"  # Location
        # "Don't know if any of this is really required-  maybe for offset plots.....?"
        n397 = property on="XY Graph" class="XYGraph (strict)"() -> ("X Scale.Range:Maximum"=w1128:dbl, "X Scale.Range:Minimum"=w1127:dbl, "Y Scale.Range:Minimum"=w1131:dbl, "Y Scale.Range:Maximum"=w1129:dbl)  [unwired: 2 in, 2 out]
        n398 = local read "Graph Height"() -> (w1139:string)
        n399 = case shown="True" w1134 {
          tunnel: w1128 -> [w1160 w1164]
          tunnel: w1127 -> [w1159 w1163]
          tunnel: [w1160 w1162] -> w1145
          tunnel: [w1159 w1161] -> w1141
          frame False {
          }
          frame True {
            n400 = Logarithm Base 10(1:w1164) -> (0:w1162:dbl)
            n401 = Logarithm Base 10(1:w1163) -> (0:w1161:dbl)
          }
        }
        n402 = case shown="True" w1137 {
          tunnel: w1129 -> [w1166 w1170]
          tunnel: w1131 -> [w1165 w1169]
          tunnel: [w1166 w1168] -> w1152
          tunnel: [w1165 w1167] -> w1130
          frame False {
          }
          frame True {
            n403 = Logarithm Base 10(1:w1169) -> (0:w1167:dbl)
            n404 = Logarithm Base 10(1:w1170) -> (0:w1168:dbl)
          }
        }
        n405 = local read "Extra range"() -> (w1132:dbl)
        n406 = Fract/Exp String To Number(string=w1139) -> (number=w1138:dbl)  [unwired: 4 out]
        n407 = Subtract(x=w1130, y=w1132) -> (x-y=w1151:dbl)
        n408 = Divide(x=0.35 ("y"), y=w1138) -> (x/y=w1150:dbl)
        n409 = Subtract(x=w1152, y=w1151) -> (x-y=w1148:dbl)
        n410 = Subtract(x=w1145, y=w1141) -> (x-y=w1144:dbl)
        n411 = Multiply(x=w1148, y=w1150) -> (x*y=w1154:dbl)
        n412 = Divide(x=w1148, y=10.0) -> (x/y=w1146:dbl)
        "Delta y" <- w1146
        n413 = Multiply(x=0.9 ("y"), y=w1144) -> (x*y=w1155:dbl)
        n414 = Multiply(x=w1144, y=-0.2 ("x")) -> (x*y=w1142:dbl)
        n415 = Subtract(x=w1151, y=w1154) -> (x-y=w1136:dbl)
        n416 = case shown="True" "Show legend?" {
          tunnel: w1136 -> [w1177 w1183]
          tunnel: [w1177 w1181] -> w1125
          tunnel: w1146 -> [_ w1184]
          frame False {
          }
          frame True {
            n417 = local read "No of Series"() -> (w1180:i32)
            n418 = Add(x=0.65, y=w1180) -> (x+y=w1179:dbl)
            n419 = Multiply(x=w1184, y=w1179) -> (x*y=w1182:dbl)
            n420 = Subtract(x=w1183, y=w1182) -> (x-y=w1181:dbl)
          }
        }
        "Y location" <- w1125
        n421 = Add(x=w1155, y=w1141) -> (x+y=w1135:dbl)
        n422 = Add(x=w1141, y=w1142) -> (x+y=→"X location":dbl)
        n423 = case shown="True" w1134 {
          tunnel: w1135 -> [w1171 w1173]
          tunnel: [w1171 w1172] -> w1123
          frame False {
          }
          frame True {
            n424 = Power Of 10(x=w1173) -> (10^x=w1172:dbl)
          }
        }
        n425 = case shown="True" w1137 {
          tunnel: w1136 -> [w1174 w1176]
          tunnel: [w1174 w1175] -> w1122
          frame False {
          }
          frame True {
            n426 = Power Of 10(x=w1176) -> (10^x=w1175:dbl)
          }
        }
        n427 = Bundle By Name(cluster=w1119, "\"At\" location.Xvalue"=w1123, "\"At\" location.Yvalue"=w1122, "Location"=w1117) -> (w1118:T9)
        n428 = call "setKey.vi"("LegendProperties"=w1118, "Set?"="Show legend?", "String in"=w1124) -> ("String out"=w1121:string)  [unwired: 7 in, 1 out]
      }
      frame "Specified Legend Position" {
        w1187 = T9 {"Appearance"={"layout"="horizontal", "text-sample order"="", "key order"="", "surroundingBox"=""}, "Alignment"={"Horizontal"="center", "Vertical"="bottom"}, "Location"="", "\"At\" location"={"XcoordSys"="", "YcoordSys"="", "Xvalue"=0.0, "Yvalue"=0.0}}  # LegendProperties
        # "Not sure if stuff below is required, to provide \"Y location\"?"
        n429 = property on="XY Graph" class="XYGraph (strict)"() -> ("Y Scale.Range:Minimum"=w1197:dbl, "Y Scale.Range:Maximum"=w1195:dbl)  [unwired: 2 in, 2 out]
        n430 = local read "Graph Height"() -> (w1203:string)
        n431 = case shown="True" w1201 {
          tunnel: w1195 -> [w1216 w1220]
          tunnel: w1197 -> [w1215 w1219]
          tunnel: [w1216 w1218] -> w1209
          tunnel: [w1215 w1217] -> w1196
          frame False {
          }
          frame True {
            n432 = Logarithm Base 10(1:w1220) -> (0:w1218:dbl)
            n433 = Logarithm Base 10(1:w1219) -> (0:w1217:dbl)
          }
        }
        n434 = local read "Extra range"() -> (w1198:dbl)
        n435 = local read "Show legend?"() -> (w1188:bool)
        n436 = Fract/Exp String To Number(string=w1203) -> (number=w1202:dbl)  [unwired: 4 out]
        n437 = Subtract(x=w1196, y=w1198) -> (x-y=w1208:dbl)
        n438 = Divide(x=0.35 ("y"), y=w1202) -> (x/y=w1207:dbl)
        n439 = local read "Legend Position"() -> (w1191:u16)
        n440 = Subtract(x=w1209, y=w1208) -> (x-y=w1206:dbl)
        n441 = property on="Legend Position" class="Ring (strict)"() -> ("Strings []"=w1192:string[])  [unwired: 2 in, 2 out]
        n442 = Multiply(x=w1206, y=w1207) -> (x*y=w1211:dbl)
        n443 = Index Array(array=w1192, index=w1191) -> (element=w1185:string)
        n444 = Divide(x=w1206, y=10.0) -> (x/y=w1204:dbl)
        n445 = Subtract(x=w1208, y=w1211) -> (x-y=w1200:dbl)
        n446 = case shown="True" w1188 {
          tunnel: w1200 -> [w1221 w1227]
          tunnel: [w1221 w1225] -> w1193
          tunnel: w1204 -> [_ w1228]
          frame False {
          }
          frame True {
            n447 = local read "No of Series"() -> (w1224:i32)
            n448 = Add(x=0.65, y=w1224) -> (x+y=w1223:dbl)
            n449 = Multiply(x=w1228, y=w1223) -> (x*y=w1226:dbl)
            n450 = Subtract(x=w1227, y=w1226) -> (x-y=w1225:dbl)
          }
        }
        n451 = Bundle By Name(cluster=w1187, "Location"=w1185) -> (w1186:T9)
        n452 = local write "Y location"(w1193) -> ()
        n453 = call "setKey.vi"("LegendProperties"=w1186, "Set?"=w1188, "String in"=w1190) -> ("String out"=w1189:string)  [unwired: 7 in, 1 out]
      }
      frame "Labels?" {
        n454 = call "setAxisGrids.vi"("Minor Gridlines"="Minor Gridlines", "Major Gridlines"="Major Gridlines", "String in"=w1232) -> ("String out"=w1231:string)  [unwired: 7 in, 1 out]
        n455 = Array Size(array="Added labels") -> (size(s)=w1240:i32)
        n456 = local read "Show Labels?"() -> (w1234:bool)
        n457 = Greater Than 0?(x=w1240) -> (x > 0?=w1236:bool)
        n458 = And(x=w1234, y=w1236) -> (x .and. y?=w1235:bool)
        n459 = Select(t="Add Labels to plot", s=w1235, f="Set plot ranges" ("t")) -> (s? t:f=w1237:string)
      }
      frame "Add Labels to plot" {
        n460 = stacked-sequence {
          seq-local: [w1255 _] -> [_ w1300]
          tunnel: [_ w1301] -> w1252
          tunnel: w1251 -> [_ w1302]
          tunnel: [_ "Set plot ranges" ("t")] -> w1248
          tunnel: w1247 -> [w1258 _]
          tunnel: w1246 -> [_ w1297]
          tunnel: w1245 -> [_ w1295]
          frame #0 {
            n461 = local read "Added labels"() -> (w1260:i32[])
            n462 = Index Array(array=w1258, index (col)=0 ("disabled index (col)")) -> (element=w1259:string[])  [unwired: 1 in]
            n463 = for {
              tunnel: w1260 -> [w1285] mode=indexing
              tunnel: w1259 -> [w1290]
              tunnel: w1258 -> [w1289]
              tunnel: "Summarise" -> [w1288]
              shift-right: [w1276] -> w1255
              shift-left: string[] [] -> [w1277]
              n464 = Add(x=w1288, y=u16 2) -> (x+y=w1286:u16)
              n465 = Index Array(array=w1289, index (col)=w1286) -> (element=w1284:string[])  [unwired: 1 in]
              n466 = Index Array(array=w1290, index=w1285) -> (element=w1281:string)
              n467 = Index Array(array=w1284, index=w1285) -> (element=w1275:string)
              n468 = call "Fast_string_Replace.vi"("Replace match with:"=" ", "Input String"=w1281, "regular expression"=":") -> ("Output String"=w1280:string)  [unwired: 2 out]
              n469 = call <vilib>:"Trim Whitespace.vi"("string"=w1280) -> ("trimmed string"=w1279:string)  [unwired: 1 in]
              n470 = Match Pattern(string=w1275, regular expression="=") -> (offset past match=w1273:i32)  [unwired: 4 out]
              n471 = Less Than 0?(x=w1273) -> (x < 0?=w1272:bool)
              n472 = Select(t="%s = %s" ("format string"), s=w1272, f="%s %s" ("format string")) -> (s? t:f=w1269:string)
              n473 = Format Into String(format string=w1269, w1279, w1275) -> (resulting string=w1262:string)  [unwired: 2 in, 1 out]
              n474 = Match Pattern(string=w1262, regular expression=";") -> (offset past match=w1267:i32)  [unwired: 4 out]
              n475 = Match Pattern(string=w1262, regular expression=" to ") -> (offset past match=w1266:i32)  [unwired: 4 out]
              n476 = Less Than 0?(x=w1267) -> (x < 0?=w1264:bool)
              n477 = Less Than 0?(x=w1266) -> (x < 0?=w1265:bool)
              n478 = And(x=w1264, y=w1265) -> (x .and. y?=w1263:bool)
              n479 = case shown="False" w1263 {
                tunnel: w1277 -> [w1291 w1294]
                tunnel: [w1291 w1292] -> w1276
                tunnel: w1262 -> [_ w1293]
                frame False {
                }
                frame True {
                  n480 = Build Array (concatenate)(w1294, w1293) -> (w1292:string[])
                }
              }
            }
          }
          frame #1 {
            n481 = local read "Show legend?"() -> (w1296:bool)
            n482 = local read "X location"() -> (w1299:dbl)
            n483 = local read "Delta y"() -> (w1298:dbl)
            n484 = for {
              shift-right: [w1323] -> w1301
              shift-left: w1302 -> [w1324]
              tunnel: w1300 -> [w1320] mode=indexing
              tunnel: w1299 -> [w1306]
              tunnel: w1298 -> [w1325]
              tunnel: w1297 -> [w1319]
              tunnel: w1296 -> [w1308]
              tunnel: w1295 -> [w1304]
              i -> [w1326]
              n485 = call "Text_for_latex.vi"("Input String"=w1320) -> ("Output String"=w1314:string)
              n486 = case shown="False" w1304 {
                tunnel: w1306 -> [w1329 w1331]
                tunnel: [w1329 w1330] -> w1305
                frame False {
                }
                frame True {
                  n487 = Power Of 10(x=w1331) -> (10^x=w1330:dbl)
                }
              }
              n488 = String Length(string=w1314) -> (length=w1317:i32)
              n489 = Less?(x=w1317, y=20) -> (x < y?=w1309:bool)
              n490 = Compound Arithmetic op=AND(w1309, invert w1308) -> (w1307:bool)
              n491 = Increment(x=w1326) -> (x+1=w1327:i32)
              n492 = case shown="True" w1307 {
                tunnel: [w1332 w1334] -> w1315
                tunnel: w1314 -> [w1332 w1335]
                tunnel: "~~~~~~~~~~~" -> [_ w1333]
                frame False {
                }
                frame True {
                  n493 = Concatenate Strings(w1333, w1335) -> (w1334:string)
                }
              }
              n494 = Multiply(x=w1326, y=w1325) -> (x*y=w1321:dbl)
              n495 = local read "Y location"() -> (w1322:dbl)
              n496 = call "Number_2_string.vi"("number"=w1305) -> ("String"=w1312:string)  [unwired: 1 in]
              n497 = Subtract(x=w1322, y=w1321) -> (x-y=w1318:dbl)
              n498 = case shown="False" w1319 {
                tunnel: w1318 -> [w1336 w1338]
                tunnel: [w1336 w1337] -> w1311
                frame False {
                }
                frame True {
                  n499 = Power Of 10(x=w1338) -> (10^x=w1337:dbl)
                }
              }
              n500 = call "Number_2_string.vi"("number"=w1311) -> ("String"=w1310:string)  [unwired: 1 in]
              n501 = Format Into String(format string="set label %d '%s' at %s, %s\n", initial string=w1324, w1327, w1315, w1312, w1310) -> (resulting string=w1323:string)  [unwired: 1 in, 1 out]
            }
          }
        }
      }
      frame "Set plot ranges" {
        w1339 = ""
        (unwired) "set border"
        (unwired) "set nologscale  y"
        (unwired) "set logscale  y"
        w1376 = "#"
        w1340 = ""
        n502 = local read "Profile offset"() -> (w1363:dbl)
        n503 = property on="XY Graph" class="XYGraph (strict)"() -> ("X Scale.Range:Maximum"=w1373:dbl, "X Scale.Range:Minimum"=w1372:dbl, "Y Scale.Range:Maximum"=w1356:dbl, "Y Scale.Range:Minimum"=w1357:dbl)  [unwired: 2 in, 2 out]
        n504 = local read "Extra range"() -> (w1367:dbl)
        n505 = Decrement(x=w1362) -> (x-1=w1364:dbl)
        n506 = Multiply(x=w1363, y=w1364) -> (x*y=w1361:dbl)
        n507 = Add(x=w1361, y=w1356) -> (x+y=w1360:dbl)
        n508 = Subtract(x=w1357, y=w1367) -> (x-y=w1368:dbl)
        n509 = call "Number_2_string.vi"("number"=w1360) -> ("String"=w1345:string)  [unwired: 1 in]
        n510 = call "Gnuplot_offset_ytics.vi"("Separation"=w1362, "Mode"="Mode", "precision"="precision", "Legend"=w1365, "Max Plot Value"=w1356, "Profile offset"=w1363) -> ("concatenated string"=w1352:string)
        n511 = call "Number_2_string.vi"("number"=w1373) -> ("String"=w1347:string)  [unwired: 1 in]
        n512 = call "Number_2_string.vi"("number"=w1372) -> ("String"=w1348:string)  [unwired: 1 in]
        n513 = call "Number_2_string.vi"("number"=w1368) -> ("String"=w1346:string)  [unwired: 1 in]
        n514 = case shown="True" w1349 {
          tunnel: [w1386 w1388] -> w1343
          tunnel: w1348 -> [w1386 _]
          tunnel: [w1385 w1387] -> w1342
          tunnel: w1347 -> [w1385 _]
          tunnel: w1346 -> [_ w1388]
          tunnel: w1345 -> [_ w1387]
          frame False {
          }
          frame True {
          }
        }
        n515 = Select(t="\nset logscale  x\n", s=w1354, f=w1340) -> (s? t:f=w1351:string)
        n516 = Select(t="\nset logscale  y\n", s=w1359, f=w1340) -> (s? t:f=w1353:string)
        n517 = case shown="\"Linear\", Default" w1344 {
          tunnel: w1343 -> [_ w1383]
          tunnel: w1342 -> [_ w1382]
          tunnel: ["" w1381] -> w1341
          frame "Spline" {
          }
          frame "Linear", Default {
            n518 = Format Into String(format string="set trange [%s : %s]", w1383, w1382) -> (resulting string=w1381:string)  [unwired: 2 in, 1 out]
          }
        }
        n519 = Format Into String(format string="%s set xrange [%s : %s] \n%s set autoscale x \n%s set yrange [%s : %s]\n%s set autoscale y\n", initial string=w1375, w1339, w1348, w1347, w1376, w1339, w1346, w1345, w1376) -> (resulting string=w1370:string)  [unwired: 1 in, 1 out]
        n520 = Concatenate Strings(w1370, w1341, w1351, w1353, w1352) -> (w1371:string)
      }
      frame "Plot Command" {
        n521 = case shown="True" w1397 {
          tunnel: ["yerrorbars" "xerrorbars"] -> w1396
          tunnel: ["" ", t"] -> w1395
          tunnel: ["t, " ""] -> w1394
          frame False {
          }
          frame True {
          }
        }
        n522 = Strip Path(path=w1409) -> (name=w1391:string)  [unwired: 1 out]
        n523 = Format Into String(format string="\nfile=\"%s.dat\"\n\nplot ", w1391) -> (resulting string=w1392:string)  [unwired: 2 in, 1 out]
        n524 = global read "Results_plotter_Global.vi" "Series Index"() -> (w1398:i32[])
        n525 = for {
          shift-right: [w1455] -> w1390
          shift-left: w1392 -> [w1456]
          tunnel: w1403 -> [w1454]
          tunnel: w1408 -> [w1449] mode=indexing
          tunnel: "Plot style" -> [w1450]
          tunnel: w1401 -> [w1437]
          tunnel: w1400 -> [w1448] mode=indexing
          tunnel: "plot error bars?" -> [w1444]
          tunnel: w1396 -> [w1427]
          tunnel: w1398 -> [w1418] mode=indexing
          tunnel: w1395 -> [w1421]
          tunnel: w1394 -> [w1420]
          i -> [w1422]
          n526 = Index Array(array=w1450, index=w1418) -> (element=w1431:u16)
          n527 = Quotient & Remainder(x=w1418, y=8) -> (x-y*floor(x/y)=w1436:i32)  [unwired: 1 out]
          n528 = call "Fast_string_Replace.vi"("Replace match with:"="", "Input String"=w1449, "regular expression"="[$]") -> ("Output String"=w1439:string)  [unwired: 2 out]
          n529 = case shown="2" w1431 {
            tunnel: ["points" ("format string") "lines" ("format string") "linespoints" ("format string")] -> w1428
            frame 0, Default {
            }
            frame 1 {
            }
            frame 2 {
            }
          }
          n530 = case shown="\"4th Poly\"" w1454 {
            tunnel: w1422 -> [_ w1466 w1479 w1486 w1493 w1501 w1508 w1515 w1522 w1529]
            tunnel: ["" w1473 w1480 w1487 w1495 w1502 w1509 w1516 w1523 w1530] -> w1453
            tunnel: w1418 -> [_ w1465 w1478 w1484 w1492 w1500 w1507 w1514 w1521 w1528]
            tunnel: 2 -> [_ w1464 w1477 w1485 w1491 w1499 w1506 w1513 w1520 w1527]
            tunnel: w1421 -> [_ _ w1475 w1483 w1489 w1497 w1504 w1511 w1518 w1525]
            tunnel: w1420 -> [_ _ w1476 w1482 w1490 w1498 w1505 w1512 w1519 w1526]
            frame "None", Default {
            }
            frame "Spline" {
              n531 = Quotient & Remainder(x=w1466, y=2) -> (x-y*floor(x/y)=w1471:i32)  [unwired: 1 out]
              n532 = Equal To 0?(x=w1471) -> (x = 0?=w1470:bool)
              n533 = Select(t="1", s=w1470, f="2") -> (s? t:f=w1467:string)
              n534 = Format Into String(format string="file index %d using 1:2 axes x1y1 linecolor %d linetype %d title '' lt %s smooth csplines, ", w1466, w1465, w1464, w1467) -> (resulting string=w1473:string)  [unwired: 2 in, 1 out]
            }
            frame "Gauss Lat" {
              n535 = Format Into String(format string="%s cmax%d*exp(-((t-offset%d)**2)/(2*sig%d**2))%s  linecolor %d linetype %d title '', ", w1476, w1479, w1479, w1479, w1475, w1478, w1477) -> (resulting string=w1480:string)  [unwired: 2 in, 1 out]
            }
            frame "Gauss vert" {
              n536 = Format Into String(format string="%s cmax%d*(exp(-((t-Zp%d)**2)/(2*sigZ%d**2))+exp(-((t+Zp%d)**2)/(2*sigZ%d**2)))%s linecolor %d linetype %d title '', ", w1482, w1486, w1486, w1486, w1486, w1486, w1483, w1484, w1485) -> (resulting string=w1487:string)  [unwired: 2 in, 1 out]
            }
            frame "Gauss Vert with 2 sig" {
              n537 = call "Vert_Spread_2_Sig.vi"("Index"=w1493) -> ("resulting string"=w1494:string)
              n538 = Format Into String(format string="%s %s%s  linecolor %d linetype %d title '', ", w1490, w1494, w1489, w1492, w1491) -> (resulting string=w1495:string)  [unwired: 2 in, 1 out]
            }
            frame "Guass glc" {
              n539 = Format Into String(format string="%s cmax%d*((t/xmax%d)**(-(1+m%d)*q%d)*exp(((1+m%d)/2)*(1-(t/xmax%d)**(-2*q%d))))%s  linecolor %d linetype %d title '', ", w1498, w1501, w1501, w1501, w1501, w1501, w1501, w1501, w1497, w1500, w1499) -> (resulting string=w1502:string)  [unwired: 2 in, 1 out]
            }
            frame "2nd Poly" {
              n540 = Format Into String(format string="%s c%d*t**2 + b%d*t + a%d%s  linecolor %d linetype %d title 'fit%d', ", w1505, w1508, w1508, w1508, w1504, w1507, w1506, w1508) -> (resulting string=w1509:string)  [unwired: 2 in, 1 out]
            }
            frame "3rd Poly" {
              n541 = Format Into String(format string="%s d%d*t**3  + c%d*t**2 + b%d*t + a%d %s linecolor %d linetype %d title 'fit%d', ", w1512, w1515, w1515, w1515, w1515, w1511, w1514, w1513, w1515) -> (resulting string=w1516:string)  [unwired: 2 in, 1 out]
            }
            frame "4th Poly" {
              n542 = Format Into String(format string="%s e%d*t**4 + d%d*t**3  + c%d*t**2 + b%d*t + a%d%s  linecolor %d linetype %d title 'fit%d', ", w1519, w1522, w1522, w1522, w1522, w1522, w1518, w1521, w1520, w1522) -> (resulting string=w1523:string)  [unwired: 2 in, 1 out]
            }
            frame "Linear" {
              n543 = Format Into String(format string="%s b%d*t + c%d%s  linecolor %d linetype %d title 'fit%d', ", w1526, w1529, w1529, w1525, w1528, w1527, w1529) -> (resulting string=w1530:string)  [unwired: 2 in, 1 out]
            }
          }
          n544 = Index Array(array=w1437, index=w1436) -> (element=w1435:i32)
          n545 = case shown="True" "Black and white?" {
            tunnel: w1418 -> [w1458 _]
            tunnel: [w1458 0] -> w1417
            frame False {
            }
            frame True {
            }
          }
          n546 = Unbundle(w1448) -> (w1447:string[])
          n547 = Array Size(array=w1447) -> (size(s)=w1446:i32)
          n548 = Greater Than 0?(x=w1446) -> (x > 0?=w1445:bool)
          n549 = And(x=w1445, y=w1444) -> (x .and. y?=w1429:bool)
          n550 = Select(t=w1427, s=w1429, f=w1428) -> (s? t:f=w1426:string)
          n551 = Select(t=":3", s=w1429, f="") -> (s? t:f=w1440:string)
          n552 = Format Into String(format string="file index %d using 1:2%s axes x1y1 title '$%s$' with ", initial string=w1456, w1422, w1440, w1439) -> (resulting string=w1443:string)  [unwired: 1 in, 1 out]
          n553 = Format Into String(format string=" linecolor %d pointtype %d pointsize %.2f linetype %d, ", initial string=w1426, w1417, w1435, "Point Size", -1) -> (resulting string=w1430:string)  [unwired: 1 in, 1 out]
          n554 = Concatenate Strings(w1443, w1430, w1453, "\\" ("string"), "\n") -> (w1455:string)
        }
        n555 = call "removeLastContinuation.vi"("String in"=w1390) -> ("String out"=w1389:string)  [unwired: 10 in]
        n556 = Concatenate Strings(w1407, w1389) -> (w1406:string)
      }
      frame "Write gnuplot file" {
        w1540 = FALSE  # append to file? (new file:F)
        w1541 = FALSE  # advisory dialog? (display:T)
        n557 = Strip Path(path=w1537) -> (stripped path=w1533:path)  [unwired: 1 out]
        n558 = Build Path(base path=w1533, name or relative path="gnuplot_script.txt") -> (appended path=w1542:path)
        n559 = call "gnuplot_legend.vi"("Plot style"=w1534, "Legend"=w1538) -> ()  [unwired: 1 out]
        n560 = call "Write_Characters_To_File.vi"("file path (dialog if empty)"=w1542, "advisory dialog? (display:T)"=w1541, "character string"=w1532, "append to file? (new file:F)"=w1540) -> ()  [unwired: 1 in, 4 out]
      }
      frame "Execute shell script" {
        n561 = call "Run_Gnuplot_Script.vi"("logfileName"=w1544, "workingDirectory"=w1545) -> ()
      }
      frame "Has pdf been generated?" {
        n562 = Strip Path(path=w1558) -> (stripped path=w1560:path, name=w1562:string)
        n563 = Concatenate Strings(w1562, ".pdf" ("string")) -> (w1561:string)
        n564 = Build Path(base path=w1560, name or relative path=w1561) -> (appended path=w1557:path)
        n565 = call "Does_file_exist_(simple).vi"("Pathname"=w1557) -> ("exists?"=w1556:bool)
        n566 = case shown="False" w1556 {
          tunnel: ["Open Standard output file" ("f") "Input Fit Coefficients into results file?"] -> w1551
          frame False {
          }
          frame True {
          }
        }
        n567 = Select(t="Show Re-Run Gnuplot?", s="Show Re-Run Gnuplot?", f=w1551) -> (s? t:f=w1552:string)
      }
      frame "Show Re-Run Gnuplot?" {
        n568 = Strip Path(path=w1569) -> (stripped path=w1568:path)  [unwired: 1 out]
        n569 = call "Re_run_Gnuplot.vi"("Plot folder (dialog if empty)"=w1568) -> ()  [unwired: 4 out]
      }
      frame "Input Fit Coefficients into results file?" {
        n570 = Greater?(x=w1579, y=T6."Spline") -> (0:w1577:bool)
        n571 = And(x="Put Coeff\nin Results file", y=w1577) -> (x .and. y?=w1575:bool)
      }
      frame "Read Fit Coefficients" {
        n572 = call "Fast_string_Replace.vi"("Replace match with:"="", "Input String"=w1592, "regular expression"=":") -> ("Output String"=w1589:string)  [unwired: 2 out]
        n573 = Strip Path(path=w1598) -> (stripped path=w1596:path)  [unwired: 1 out]
        n574 = Build Path(base path=w1596, name or relative path="Coeff.txt") -> (appended path=w1595:path)
        n575 = call "Read_File_Simple.vi"("Filename"=w1595) -> ("string"=w1593:string)  [unwired: 2 in, 7 out]
        n576 = for {
          tunnel: w1594 -> [w1616]
          tunnel: w1593 -> [w1613]
          tunnel: w1589 -> [w1612]
          tunnel: [w1610] -> w1588
          tunnel: w1587 -> [w1609] mode=indexing
          shift-right: [w1605] -> w1585
          shift-left: string[][] [] -> [w1606]
          i -> [w1615]
          n577 = case shown="\"Gauss vert\"" w1616 {
            tunnel: w1615 -> [_ w1637 w1641 w1657]
            tunnel: [string[] [] w1633 w1649 w1663] -> w1614
            tunnel: [string[] [] w1629 w1646 w1660] -> w1611
            frame "None", Default {
            }
            frame "Gauss Lat" {
              n578 = Format Into String(format string="sig%d", w1637) -> (resulting string=w1635:string)  [unwired: 2 in, 1 out]
              n579 = Format Into String(format string="offset%d", w1637) -> (resulting string=w1634:string)  [unwired: 2 in, 1 out]
              n580 = Format Into String(format string="cmax%d", w1637) -> (resulting string=w1636:string)  [unwired: 2 in, 1 out]
              n581 = Build Array(":Max:Lat", ":Sig Y:", ":Yo:") -> (w1629:string[])
              n582 = Build Array(w1636, w1635, w1634) -> (w1633:string[])
            }
            frame "Gauss Vert with 2 sig" {
              n583 = Format Into String(format string="Zp%d", w1641) -> (resulting string=w1650:string)  [unwired: 2 in, 1 out]
              n584 = Format Into String(format string="cmax%d", w1641) -> (resulting string=w1652:string)  [unwired: 2 in, 1 out]
              n585 = Format Into String(format string="sigZ_low%d", w1641) -> (resulting string=w1642:string)  [unwired: 2 in, 1 out]
              n586 = Format Into String(format string="sigZ_up%d", w1641) -> (resulting string=w1651:string)  [unwired: 2 in, 1 out]
              n587 = Build Array(":Max:Vert", ":Sig Z:Upper", ":Sig Z:Lower", ":Zp:") -> (w1646:string[])
              n588 = Build Array(w1652, w1651, w1642, w1650) -> (w1649:string[])
            }
            frame "Gauss vert" {
              n589 = Format Into String(format string="Zp%d", w1657) -> (resulting string=w1664:string)  [unwired: 2 in, 1 out]
              n590 = Format Into String(format string="cmax%d", w1657) -> (resulting string=w1665:string)  [unwired: 2 in, 1 out]
              n591 = Format Into String(format string="sigZ%d", w1657) -> (resulting string=w1656:string)  [unwired: 2 in, 1 out]
              n592 = Build Array(":Max:Vert", ":Sig Z:Upper", ":Sig Z:Lower", ":Zp:") -> (w1660:string[])
              n593 = Build Array(w1665, w1656, w1656, w1664) -> (w1663:string[])
            }
          }
          n594 = Unbundle(w1609) -> ("Output"=w1603:dbl[])  [unwired: 1 out]
          n595 = for {
            tunnel: w1614 -> [w1626] mode=indexing
            tunnel: w1613 -> [w1623]
            tunnel: [w1621] -> w1608 mode=indexing
            n596 = Concatenate Strings(w1626, " = " ("string")) -> (w1624:string)
            n597 = Match Pattern(string=w1623, regular expression=w1624) -> (after substring=w1622:string)  [unwired: 4 out]
            n598 = call "Split_at_return.vi"("String"=w1622) -> ("before substring"=w1621:string)  [unwired: 1 in, 3 out]
          }
          n599 = for {
            tunnel: w1612 -> [w1620]
            tunnel: w1611 -> [w1619] mode=indexing
            tunnel: [w1618] -> w1610 mode=indexing
            n600 = Concatenate Strings(w1620, w1619) -> (w1618:string)
          }
          n601 = Array Size(array=w1603) -> (size(s)=w1604:i32)
          n602 = for {
            N: w1604 -> [_]
            tunnel: w1608 -> [w1617]
            tunnel: [w1617] -> w1607 mode=indexing
          }
          n603 = Build Array (concatenate)(w1606, w1607) -> (w1605:string[][])
        }
        n604 = global write "Results_plotter_Global.vi" "New Chs In"(w1588) -> ()
        n605 = global write "Results_plotter_Global.vi" "New Values In"(w1585) -> ()
      }
      frame "Open Standard output file" {
        n606 = Strip Path(path=w1673) -> (stripped path=w1670:path)  [unwired: 1 out]
        n607 = Format Into String(format string="open \"%s\"", w1671) -> (resulting string=w1669:string)  [unwired: 2 in, 1 out]
        n608 = call <vilib>:"System Exec.vi"("working directory"=w1670, "command line"=w1669) -> ()  [unwired: 4 in, 6 out]
      }
    }
  }
  "Tex Info String" <- w17
  "Saved Automatically?" <- FALSE
